vi "eyecat MAX v2_JS.vi"() -> ()   [LabVIEW 2014]
doc: "This VI is an upgrade from the WIN 1_v4 that implements the ageing subrutine"
uses:
  <vilib>/Utility/file.llb/Write To Spreadsheet File (string).vi
  <vilib>/Utility/file.llb/Read From Spreadsheet File (string).vi
  <vilib>/regexp/Match Regular Expression.xnode
  Controls Win/Control 3.ctl
  <vilib>/Utility/miscctls.llb/LVRowAndColumnTypeDef.ctl
  <vilib>/Platform/TimedLoop/XDataNode/XDataNode.xnode
  <vilib>/Platform/TimedLoop/XDataNode/nitl_modes.ctl
  <vilib>/Platform/TimedLoop/XDataNode/XDNodeRunTimeDep.lvlib
  <vilib>/Platform/TimedLoop/XDataNode/wakeup.ctl
  <vilib>/Platform/TimedLoop/XDataNode/timing_clust.ctl
  Buttons/Numeric control.ctl
  <vilib>/Utility/file.llb/Read From Spreadsheet File (DBL).vi
  Buttons/String input.ctl
  Buttons/Numeric indicator.ctl
  Buttons/String output.ctl
panel:
  in  "7170 Override":bool
  out "NO":dbl[](array[numeric])
  out "CO":dbl[](array[numeric])
  out "MKS":bool
  out "7170":bool
  out "Pressure":dbl
  in  "Duration -1":i32
  in  "Demo Sync":i32
  in  "Demo On":bool
  in  "FlowGuide":bool
  in  "Mean(Off)/Interval(On) 2":bool
  in  "Flow Band %":dbl=1.04
  in  "Flow Sync":i32
  in  "Execute Leak Test Button":bool
  out "Emissions":dbl[](array[numeric])
  in  "Temperature Sync":i32
  in  "TempGuide":bool
  in  "Temp Band %":dbl=1.04
  in  "Mean(Off)/Interval(On)":bool
  in  "MKS 5Hz":bool
  out "output cluster":T2
  out "Lambda":dbl[](array[numeric])
  out "MKS HC":dbl
  in  "HC Index":i32
  in  "MFC Number":i32
  out "Open/Closed \nLoop":dbl[](array[numeric])
  out "Air Cyc 2":dbl[](array[numeric])
  in  "Cycle size":i32
  out "MFC Setpoint/Delivery":dynamicdata(graph)
  out "ExtAnDn":bool
  out "ExtAnUp":bool
  out "HC Cyc 2":dbl[](array[numeric])
  out "SO Valve 2":dbl[](array[numeric])
  out "SO Valve 1":dbl[](array[numeric])
  out "Air Bal":dbl[](array[numeric])
  out "HC Bal":dbl[](array[numeric])
  out "Air Cyc 1":dbl[](array[numeric])
  out "HC Cyc 1":dbl[](array[numeric])
  out "File name":string
  out "Log?":bool
  out "Advanced Logging":bool
  out "Connected":bool
  out "Furnace temp 2":dbl
  out "Full system?":bool
  out "Log interval (seconds)":T1
  in  "Flow rate Age":dbl
  in  "Inlet temp Age":dbl
  out "Stopped?":bool
  in  "Stop Cmd":T1
  out "Connected?":bool
  out "Error":dbl
  out "Iteration Duration":i64
  out "Finished Late? [i-1]":bool
  out "Furnace temp 1":dbl
  out "stop 2":bool
  in  "Enum 1":i16=1
  in  "Acknowledge":bool
  out "Test number":u16
  out "Flag1":bool=TRUE
  out "EditPos Subc":T3
  out "Flag 2":bool=TRUE
  in  "Tab Control":T4(tab)
  in  "Leak Test":bool
  in  "Stop Test":bool
  in  "Log Test Data":bool
  in  "Start Test":bool
  in  "Adv Settings":bool
  out "Doors Unlocked":bool
  in  "Temperature Limit (°C)":T1=800.0 min=0.0 max=1200.0 step=1.0
  in  "File Name":T5="Test"
  in  "File Path":path=path "C:/DATA LOG"
  out "Fail":bool
  out "Pass":bool
  in  "Select Test Type":T6(radio)
  out "Standby":bool
  out "Doors Open":bool
  out "Extractor Fan On":bool
  out "Test In Progress":bool
  out "Cool Down":bool
  out "System Alarm":bool
  in  "Inlet Temperature (°C)":T1=400.0 min=350.0 max=1000.0 step=1.0
  in  "Inlet LAMBDA Rich":T1=0.9 min=0.85 max=0.96 step=0.001
  in  "Inlet LAMBDA Lean":T1=1.2 min=1.02 max=3.0 step=0.001
  in  "Test Stop temperature (°C)":T1=300.0 min=100.0 max=1000.0 step=1.0
  in  "Test Start Temperature (°C)":T1=125.0 min=0.0 max=500.0 step=1.0
  in  "Furnace Ramp Rate (°C/min)":T1=15.0 min=1.0 max=50.0 step=0.1
  in  "NO:CO Ratio":T1=1.1 min=1.0 max=5.0 step=0.1
  in  "Inlet O2 (%)":T1=0.5 min=0.0 max=14.0 step=0.01
  in  "Inlet LAMBDA":T1=1.0 min=0.6 max=3.0 step=0.001
  out "Space Velocity (h-1)":T7
  out "Vol Flow @ STP (l/min)":T7
  in  "Test Flow Rate(g/s)":T1 min=0.0 max=100.0 step=0.01
  out "Sample Volume (litres)":T7
  in  "Number of Samples":T1=1.0 min=1.0 max=6.0 step=1.0
  in  "Sample Diameter (mm)":T1
  out "CO Theory (%)":T7 format="%#_3g"
  out "CO Theory (%)":T7 format="%#_3g"
  out "HC Theory (%)":T7
  in  "Sample Length (mm)":T1 min=0.0 step=0.5
  in  "NO ppm SW":dbl=500.0 caption="NO (ppm)" min=0.0 max=500.0 step=1.0
  in  "NO ppm Loff":T1 caption="NO ppm"
  in  "Delete sCycle":bool
  in  "Load sCycle":bool
  in  "Save sCycle":bool
  in  "Clear subcycle":bool
  in  "Clear Cycle Pattern":bool
  in  "Save Cycle":bool
  in  "Load Cycle":bool
  in  "Delete Cycle":bool
  out "Test Compiled":bool
  in  "Compile Test Button":bool
  in  "Sub-Cycle List":i32(listbox)=1
  in  "Cycle List":i32(listbox)=2
  out "Total Test Duration (hrs)":T8
  in  "Ageing Gas":enum32{"Radio Selection 1", "Radio Selection 2"}(radio)
  in  "Sub-Cycle Pattern":string[][](table) caption="Subcycle pattern"
  in  "Total Number of Cycles":T1=1.0 min=1.0 max=10000.0 step=1.0
  in  "Cycle Pattern":string[][](table)
  in  "Sub-Cycle Name":T5
  in  "Cycle Name":T5
  out "Heat Exchanger Temperatures (°C)":dynamicdata(graph)
  out "Flow Rate (g/s)":dynamicdata(graph)
  out "Sample Temperatures (°C)":dynamicdata(graph)
  out "System Temperatures (°C)":dynamicdata(graph)
  out "HC Concentration (ppm)":dynamicdata(graph)
  out "Lambda":dynamicdata(graph)
  out "O2/CO Concentration":dynamicdata(graph)
  out "NO Concentration (ppm)":dynamicdata(graph)
  in  "Purge System":bool
  in  "Alarm ack":bool
  in  "Clear log":bool
  out "Table":string[][](table)
  out "Soft Alarm":bool
  out "Hard Alarm":bool
  # "0 CO \n1 HC Cyc 1\n2 Air Cyc 1\n3 NO\n4 Air Bal\n5 HC Bal\n6 Air Cyc 2\n7 HC Cyc 2"
  # "1% = 0.01"
  # "Test Type"
  # "Test Commands"
  # "System Indicators"
  # "Leak Test"
  # "Catalyst Specification"
  # "Lightoff Settings"
  # "Furnace Lightoff Settings"
  # "Sweep Settings"
  # "CO/HC Lightoff Settings"
  # "0.96 < lambda < 0.85"
  # "1.02< lambda < 1.6"
  # "350 < Tinlet < 1000"
  # "NO Lightoff Settings"
  # "Flow Specification"
  # "Cycle Compiled"
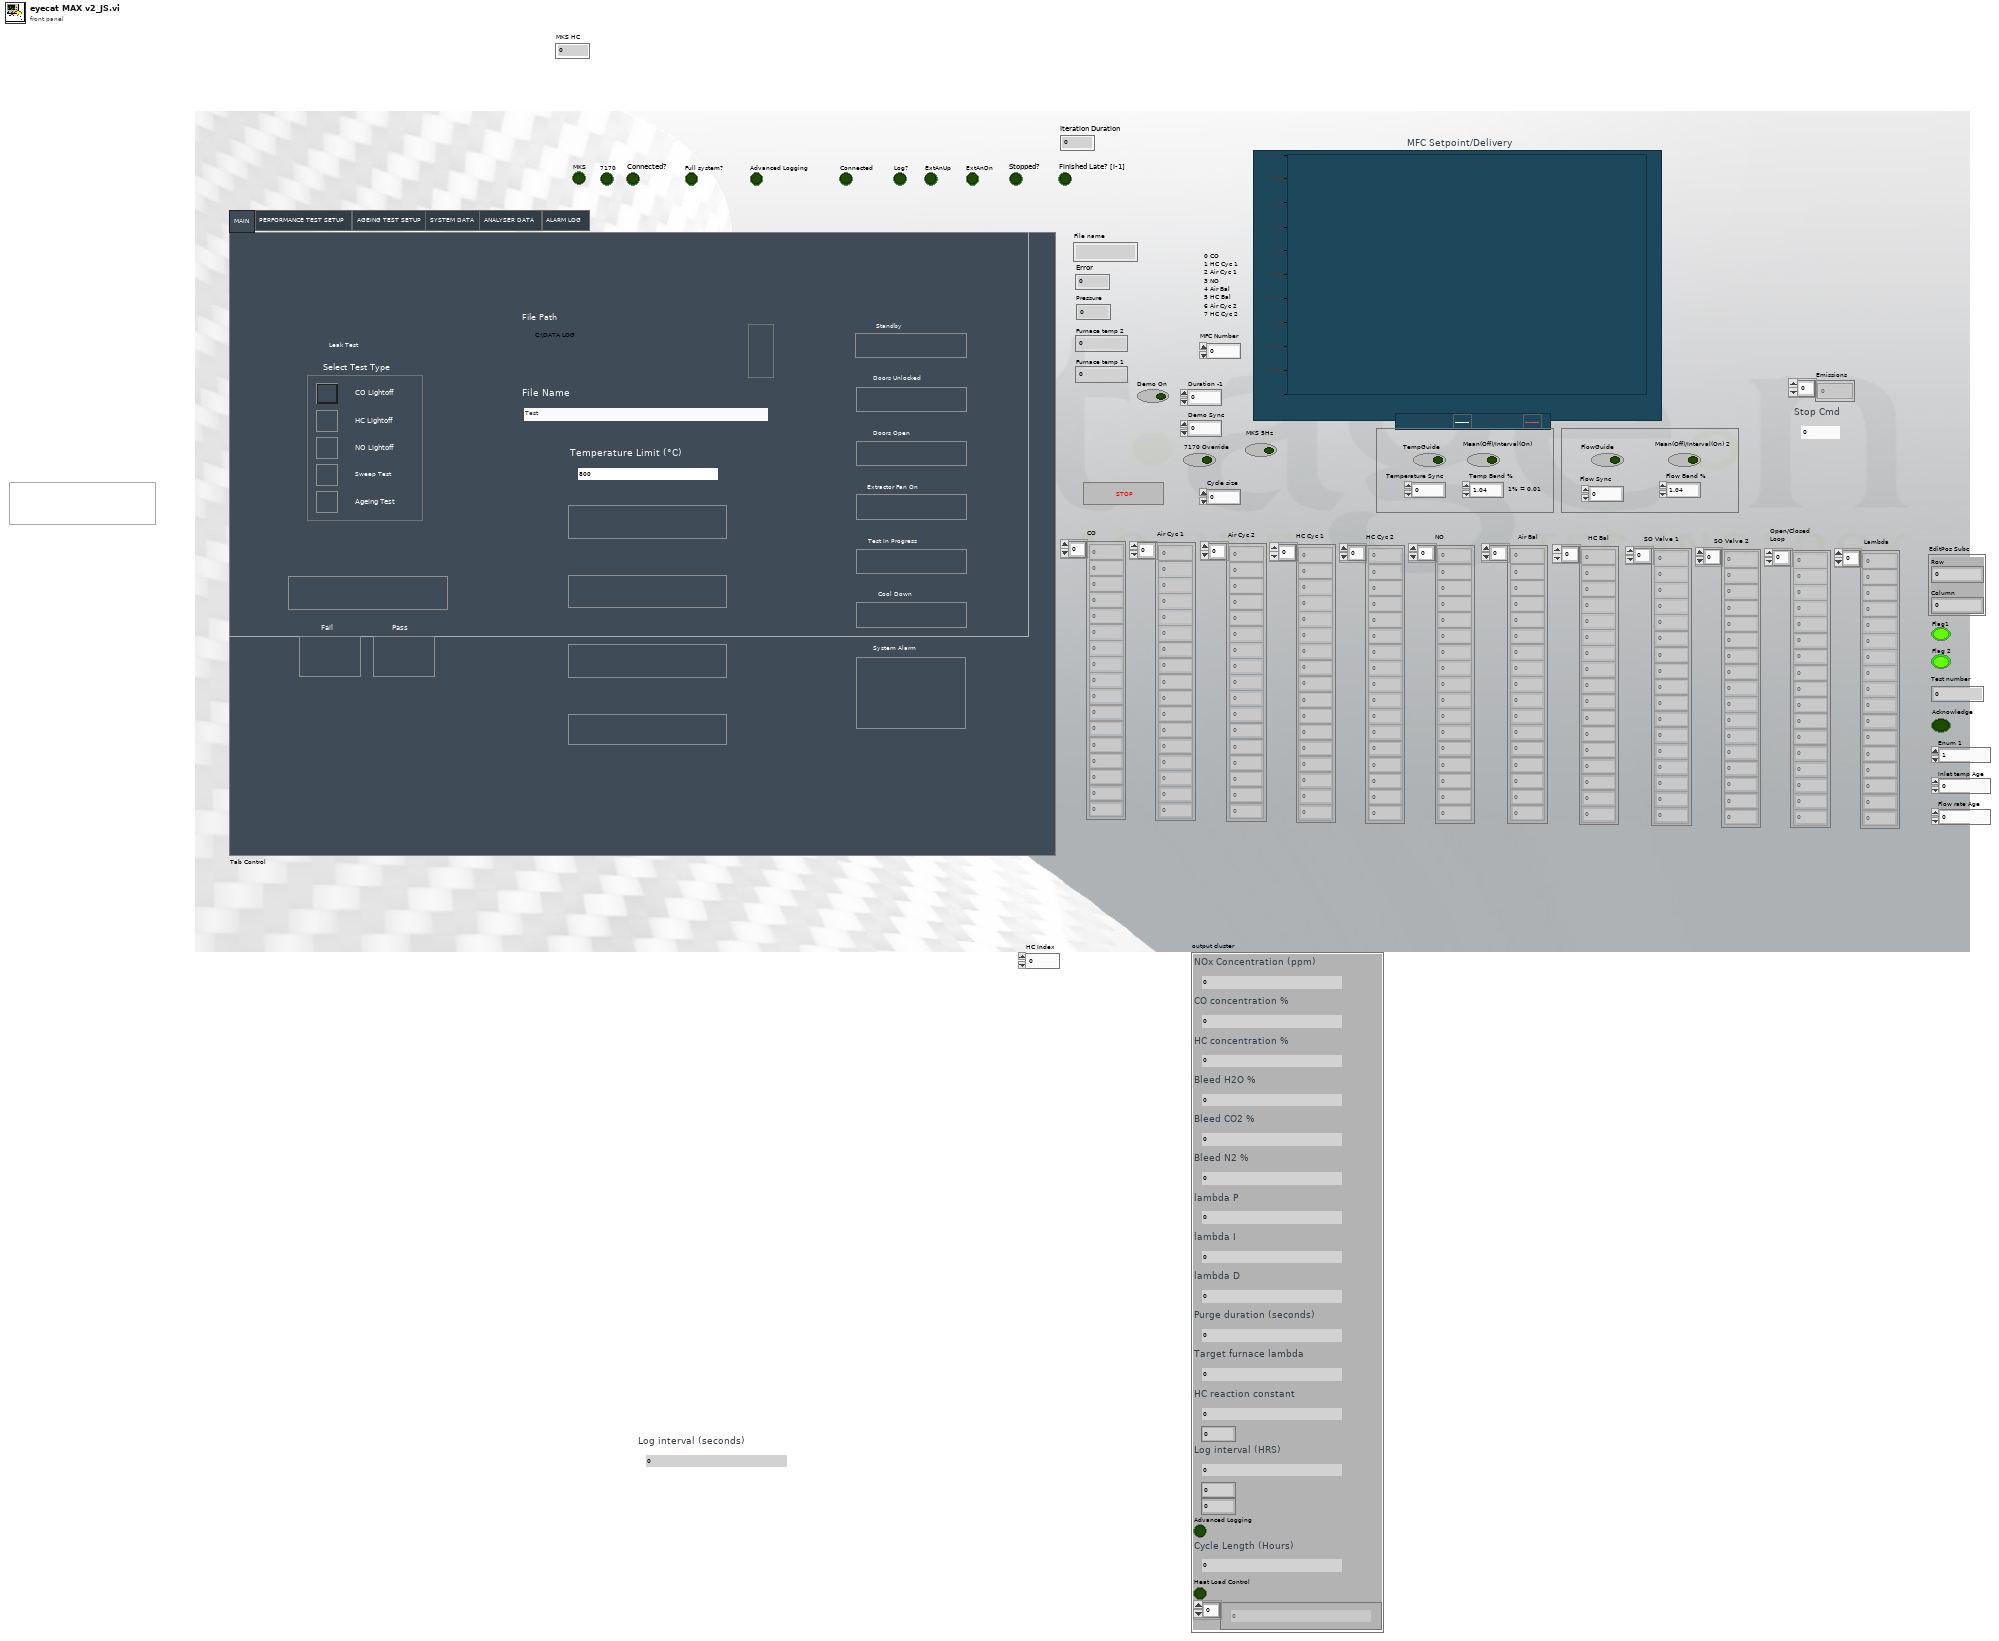
[diagram p1: front panel]
types:
  T1 = typedef "Numeric control.ctl" = dbl
  T2 = cluster{"NOx Concentration (ppm)":T1, "CO concentration %":T1, "HC concentration %":T1, "Bleed H2O %":T1, "Bleed CO2 %":T1, "Bleed N2 %":T1, "lambda P":T1, "lambda I":T1, "lambda D":T1, "Purge duration (seconds)":T1, "Target furnace lambda":T1, "HC reaction constant":T1, i16, "Log interval (HRS)":T1, i16, i16, "Advanced Logging":bool, "Cycle Length (Hours)":T1, "Heat Load Control":bool, T1[]}
  T3 = typedef "LVRowAndColumnTypeDef.ctl" = cluster{"Row":i32, "Column":i32}
  T4 = enum32{"MAIN", "PERFORMANCE TEST SETUP", "AGEING TEST SETUP", "SYSTEM DATA", "ANALYSER DATA", "ALARM LOG"}
  T5 = typedef "String input.ctl" = string
  T6 = enum32{"CO Lightoff", "HC Lightoff", "NO Lightoff", "Sweep Test", "Ageing Test"}
  T7 = typedef "Numeric indicator.ctl" = dbl
  T8 = typedef "String output.ctl" = string
  T9 = typedef "XDNodeRunTimeDep.lvlib/nitl_modes.ctl" = enum32{"No Change", "Process missed periods, maintain original phase", "Discard missed periods, maintain original phase", "Process missed periods, ignore original phase", "Discard missed periods, ignore original phase"}
  T10 = typedef "Control 3.ctl" = enum16{"main", "start test", "save subc", "load subc", "delete subc", "clear table 1", "update list 1", "save cycle", "load cycle", "delete cycle", "clear table 2", "update list 2", "calc HC CO", "Total time calc", "update Cycle pattern ", "load cycle name", "convert to num", "load test array", "check scycle name", "check cycle name", "Multigas connect", "Multigas disconnect", "Leak Test"}
  T11 = enum8{"Enabled", "Disabled", "Disabled and Grayed Out"}
  T12 = typedef "XDNodeRunTimeDep.lvlib/timing_clust.ctl" = cluster{"Expected End [f-1]":u64, "Actual End [f-1]":u64, "Finished Late? [f-1]":bool, "Expected End [i-1]":u64, "Actual End [i-1]":u64, "Finished Late? [i-1]":bool, "Expected Start [i]":u64, "Actual Start [i]":u64, "Expected Start [f]":u64, "Actual Start [f]":u64, "Source Name":string, "Structure Name":string, "Period":i64, "Deadline":i64, "Offset":i64, "Start":i64, "Priority":i32, "Timeout":i32, "Mode":T9, "Wakeup Reason":T13, "Error":errorcluster, "Source Type":string, "Secondary Source Type":string, "Global End Time":u64, "Global Start Time":u64, "Frame Duration":u64, "Iteration Duration":u64, "Assigned CPU":i32, "I/O Scan Engine Mode":u32}
  T13 = typedef "XDNodeRunTimeDep.lvlib/wakeup.ctl" = enum32{"Normal", "Aborted", "Asynchronous wakeup", "Timing source error", "Timed loop error", "Timeout"}
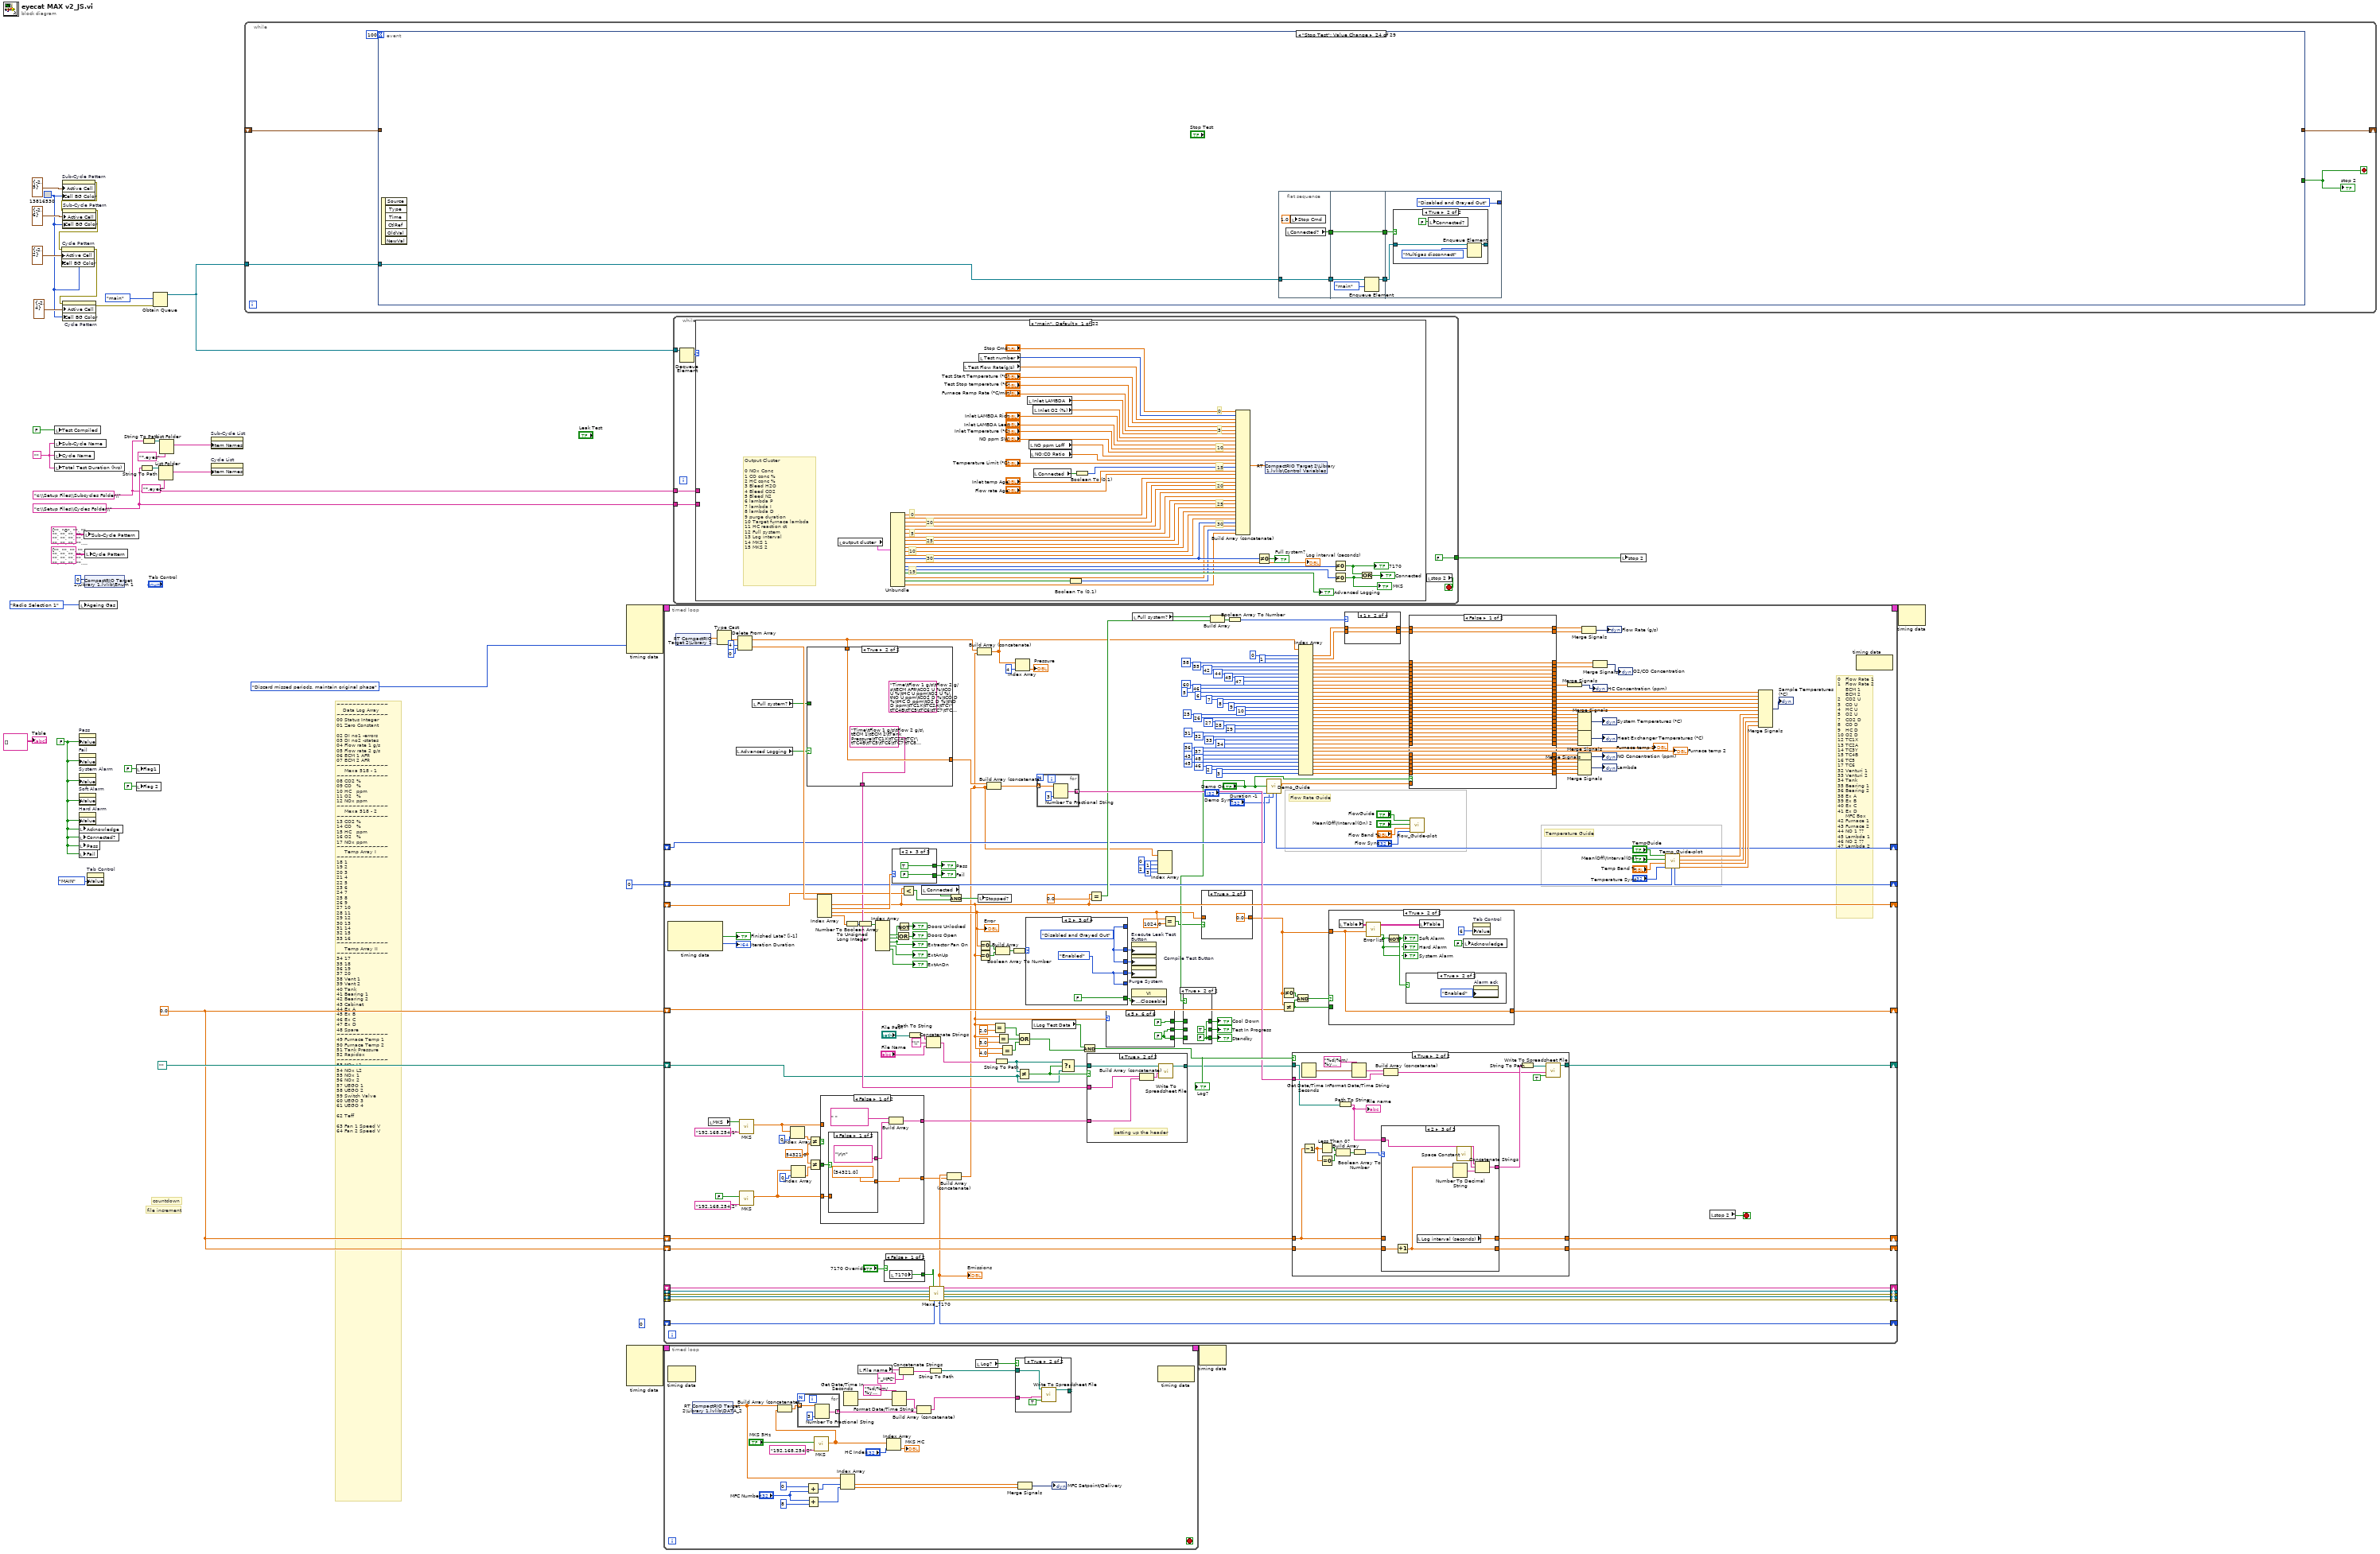
[diagram p0: block diagram]
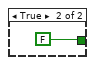
[diagram p3: hidden frame]
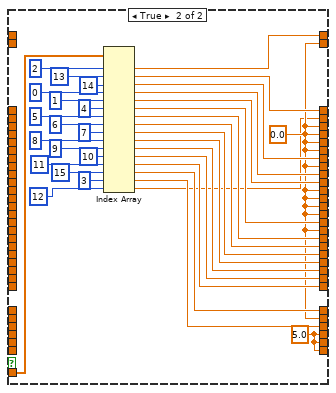
[diagram p6: hidden frame]
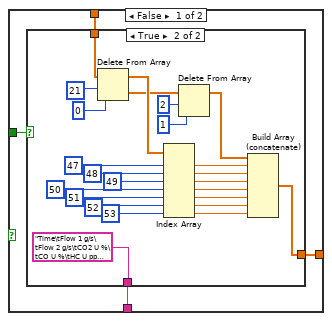
[diagram p7: hidden frame]
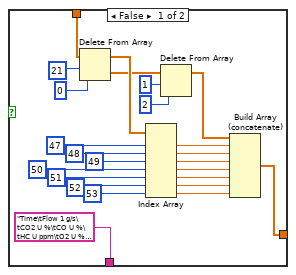
[diagram p8: hidden frame]
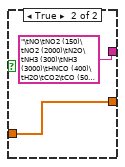
[diagram p9: hidden frame]
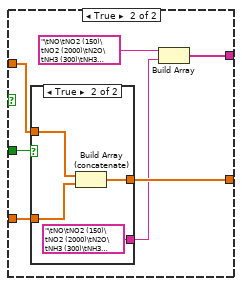
[diagram p10: hidden frame]
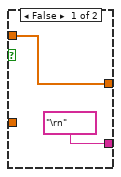
[diagram p11: hidden frame]
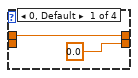
[diagram p12: hidden frame]
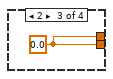
[diagram p13: hidden frame]
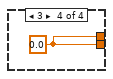
[diagram p14: hidden frame]
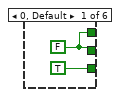
[diagram p15: hidden frame]
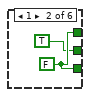
[diagram p16: hidden frame]
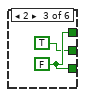
[diagram p17: hidden frame]
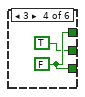
[diagram p18: hidden frame]
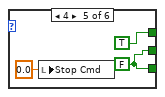
[diagram p19: hidden frame]
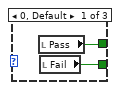
[diagram p20: hidden frame]
diagram:
  (unwired) 0 ("index")
  w5 = FALSE
  w4 = 0.0 ("y")
  w21 = ""
  w24 = "c:\\Setup Files\\Cycles Folder\\"
  w30 = u32 13816530
  w22 = "c:\\Setup Files\\Subcycles Folder\\"
  # "~~~~~~~~~~~~~\n    Data Log Array\n~~~~~~~~~~~~~\n00 Status Integer\n01 Zero Constant\n\n02 DI no1 -errors\n03 DI no2 -states\n04 Flow rate 1 g/s\n05 Flow rate 2 g/s\n06 ECM 1 AFR\n07 ECM 2 AFR\n~~~~~~~~~~~~~\n     Mexa 518 - 1\n~~~~~~~~~~~~~\n08 CO2 %\n09 CO   %\n10 HC   ppm\n11 O2   %\n12 NOx ppm\n~~~~~~~~~~~~~\n     Mexa 518 - 2\n~~~~~~~~~~~~~\n13 CO2 %\n14 CO   %\n15 HC   ppm\n16 O2   %\n17 NOx ppm\n~~~~~~~~~~~~~\n     Temp Array I\n~~~~~~~~~~~~~\n18 1\n19 2 \n20 3\n21 4\n22 5\n23 6\n24 7\n25 8\n26 9\n27 10\n28 11\n29 12\n30 13\n31 14\n32 15\n33 16\n~~~~~~~~~~~~~\n     Temp Array II\n~~~~~~~~~~~~~\n34 17\n35 18\n36 19\n37 20\n38 Vent 1\n39 Vent 2\n40 Tank\n41 Bearing 1\n42 Bearing 2\n43 Cabinet\n44 Ex A\n45 Ex B\n46 Ex C\n47 Ex D\n48 Spare\n~~~~~~~~~~~~~\n49 Furnace Temp 1\n50 Furnace Temp 2\n51 Tank Pressure\n52 Rapidox\n~~~~~~~~~~~~~\n53 NOx L1\n54 NOx L2\n55 NOx 1\n56 NOx 2\n57 UEGO 1\n58 UEGO 2\n59 Switch Valve\n60 UEGO 3\n61 UEGO 4\n\n62 Teff\n\n63 Fan 1 Speed V\n64 Fan 2 Speed V"
  # "file increment"
  # "countdown"
  n1 = local write "Test Compiled"(FALSE ("Cycle Compiled")) -> ()
  n2 = local write "Sub-Cycle Name"(w21) -> ()
  n3 = local write "Cycle Name"(w21) -> ()
  n4 = local write "Total Test Duration (hrs)"(w21) -> ()
  n5 = property on="Sub-Cycle Pattern" class="Tbl (strict)"("Active Cell"=T3 {"Row"=-2, "Column"=5} ("Active Cell:Active Cell"), "Cell BG Color"=w30) -> (error out=w35:errorcluster)  [unwired: 2 in, 1 out]
  n6 = property on="Sub-Cycle Pattern" class="Tbl (strict)"(error in=w35, "Active Cell"=T3 {"Row"=-2, "Column"=6} ("Active Cell:Active Cell"), "Cell BG Color"=w30) -> (error out=w34:errorcluster)  [unwired: 1 in, 1 out]
  n7 = property on="Cycle Pattern" class="Tbl (strict)"(error in=w34, "Active Cell"=T3 {"Row"=-2, "Column"=2} ("Active Cell:Active Cell"), "Cell BG Color"=w30) -> (error out=w32:errorcluster)  [unwired: 1 in, 1 out]
  n8 = property on="Cycle Pattern" class="Tbl (strict)"(error in=w32, "Active Cell"=T3 {"Row"=-2, "Column"=4} ("Active Cell:Active Cell"), "Cell BG Color"=w30) -> (error out=w29:errorcluster)  [unwired: 1 in, 1 out]
  n9 = property on="Pass" class="Bool (strict)"("Value"=w5) -> ()  [unwired: 2 in, 2 out]
  n10 = property on="Fail" class="Bool (strict)"("Value"=w5) -> ()  [unwired: 2 in, 2 out]
  n11 = property on="System Alarm" class="Bool (strict)"("Value"=w5) -> ()  [unwired: 2 in, 2 out]
  n12 = property on="Soft Alarm" class="Bool (strict)"("Value"=w5) -> ()  [unwired: 2 in, 2 out]
  n13 = property on="Hard Alarm" class="Bool (strict)"("Value"=w5) -> ()  [unwired: 2 in, 2 out]
  n14 = local write "Acknowledge"(w5) -> ()
  n15 = local write "Connected?"(w5) -> ()
  n16 = local write "Pass"(w5) -> ()
  n17 = local write "Fail"(w5) -> ()
  n18 = local write "Ageing Gas"(enum32{"Radio Selection 1", "Radio Selection 2"}."Radio Selection 1" ("Ageing Gas")) -> ()
  n19 = local write "Sub-Cycle Pattern"(string[][] [["", "0", "", "", "", "", "", "", "", "", "", "", ""], ["", "", "", "", "", "", "", "", "", "", "", "", ""], ["", "", "", "", "", "", "", "", "", "", "", "", ""], ["", "", "", "", "", "", "", "", "", "", "", "", ""], ["", "", "", "", "", "", "", "", "", "", "", "", ""], ["", "", "", "", "", "", "", "", "", "", "", "", ""], ["", "", "", "", "", "", "", "", "", "", "", "", ""], ["", "", "", "", "", "", "", "", "", "", "", "", ""], ["", "", "", "", "", "", "", "", "", "", "", "", ""], ["", "", "", "", "", "", "", "", "", "", "", "", ""], ["", "", "", "", "", "", "", "", "", "", "", "", ""], ["", "", "", "", "", "", "", "", "", "", "", "", ""], ["", "", "", "", "", "", "", "", "", "", "", "", ""], ["", "", "", "", "", "", "", "", "", "", "", "", ""], ["", "", "", "", "", "", "", "", "", "", "", "", ""], ["", "", "", "", "", "", "", "", "", "", "", "", ""], ["", "", "", "", "", "", "", "", "", "", "", "", ""], ["", "", "", "", "", "", "", "", "", "", "", "", ""], ["", "", "", "", "", "", "", "", "", "", "", "", ""], ["", "", "", "", "", "", "", "", "", "", "", "", ""], ["", "", "", "", "", "", "", "", "", "", "", "", ""], ["", "", "", "", "", "", "", "", "", "", "", "", ""], ["", "", "", "", "", "", "", "", "", "", "", "", ""], ["", "", "", "", "", "", "", "", "", "", "", "", ""], ["", "", "", "", "", "", "", "", "", "", "", "", ""], ["", "", "", "", "", "", "", "", "", "", "", "", ""], ["", "", "", "", "", "", "", "", "", "", "", "", ""], ["", "", "", "", "", "", "", "", "", "", "", "", ""], ["", "", "", "", "", "", "", "", "", "", "", "", ""], ["", "", "", "", "", "", "", "", "", "", "", "", ""], ["", "", "", "", "", "", "", "", "", "", "", "", ""]]) -> ()
  n20 = local write "Cycle Pattern"(string[][] [["", "", "", "", ""], ["", "", "", "", ""], ["", "", "", "", ""], ["", "", "", "", ""], ["", "", "", "", ""], ["", "", "", "", ""], ["", "", "", "", ""], ["", "", "", "", ""], ["", "", "", "", ""], ["", "", "", "", ""], ["", "", "", "", ""], ["", "", "", "", ""], ["", "", "", "", ""], ["", "", "", "", ""], ["", "", "", "", ""], ["", "", "", "", ""], ["", "", "", "", ""], ["", "", "", "", ""], ["", "", "", "", ""], ["", "", "", "", ""], ["", "", "", "", ""], ["", "", "", "", ""], ["", "", "", "", ""], ["", "", "", "", ""], ["", "", "", "", ""], ["", "", "", "", ""], ["", "", "", "", ""], ["", "", "", "", ""], ["", "", "", "", ""], ["", "", "", "", ""], ["", "", "", "", ""]]) -> ()
  n21 = shared-variable "RT CompactRIO Target 2\\Library 1.lvlib\\Enum 1"(u16 0 ("Enum 1")) -> ()  [unwired: 1 in, 1 out]
  n22 = property on="Tab Control" class="TabCtl (strict)"("Value"=T4."MAIN" ("Tab Control")) -> ()  [unwired: 2 in, 2 out]
  n23 = local write "Flag1"(FALSE) -> ()
  n24 = local write "Flag 2"(FALSE) -> ()
  n25 = String To Path(string=w24) -> (path=w25:path)
  n26 = String To Path(string=w22) -> (path=w27:path)
  n27 = Obtain Queue(element data type=Control_3."main" ("Enum"), error in (no error)=w29) -> (queue out=w38:refnum<queue>)  [unwired: 3 in, 2 out]
  n28 = List Folder(path=w25, pattern="*.eyec") -> (filenames=w26:string[])  [unwired: 2 in, 3 out]
  n29 = List Folder(path=w27, pattern="*.eyes") -> (filenames=w28:string[])  [unwired: 2 in, 3 out]
  n30 = property on="Sub-Cycle List" class="LstBox (strict)"("Item Names"=w28) -> ()  [unwired: 2 in, 2 out]
  n31 = property on="Cycle List" class="LstBox (strict)"("Item Names"=w26) -> ()  [unwired: 2 in, 2 out]
  n32 = while {
    tunnel: w38 -> [w44]
    shift-right: [w42] -> _
    shift-left: _ -> [w41]
    stop <- w40 stop-if-true
    n33 = event shown="[23] \"Stop Test\": Value Change" {
      selector: _ -> [_ _ _ _ _ _ _ _ _ _ _ _ _ _ _ _ _ _ _ _ _ _ _ _ _ _ _ _ _]
      dyn-events: _ -> [_ _ _ _ _ _ _ _ _ _ _ _ _ _ _ _ _ _ _ _ _ _ _ _ _ _ _ _ _]
      timeout: 100 -> [_ _ _ _ _ _ _ _ _ _ _ _ _ _ _ _ _ _ _ _ _ _ _ _ _ _ _ _ _]
      tunnel: w44 -> [w47 w49 _ w58 w66 w73 w80 w91 w95 w106 w111 w114 w119 w141 w149 w150 _ _ _ _ w195 w211 _ w297 w315 _ w329 _ _]
      tunnel: [w45 w48 _ w59 w65 w72 w79 w90 w93 w101 w108 w113 w117 w138 _ _ _ _ _ _ _ _ _ _ _ _ _ _ _] -> w42
      tunnel: w41 -> [w45 w48 _ w59 w65 w72 w78 w90 w93 w101 w108 w113 w117 w138 _ _ _ _ _ _ _ _ _ _ _ _ _ _ _]
      tunnel: [_ _ w51 _ _ _ _ _ _ _ _ _ _ _ _ _ _ _ _ _ _ _ _ _ _ _ _ _ _] -> w40
      event Timeout {
        n34 = event-data() -> ()  [unwired: 1 in, 2 out]
        n35 = Enqueue Element(queue=w47, element=Control_3."main" ("Enum")) -> ()  [unwired: 2 in, 3 out]
      }
      event "Clear subcycle": Value Change {
        n36 = event-data() -> ()  [unwired: 1 in, 5 out]
        n37 = Enqueue Element(queue=w49, element=Control_3."clear table 1" ("Enum")) -> ()  [unwired: 2 in, 3 out]
      }
      event Panel Close? {
        n38 = event-data() -> ()  [unwired: 1 in, 3 out]
        n39 = Two Button Dialog(message="This command will close Eyecat!\nDo you wish to continue?", 1:"No" ("F button name (\"Cancel\")"), 2:"Yes" ("T button name (\"OK\")")) -> (T button?=w51:bool)
        n40 = Not(x=w51) -> (.not. x?=w52:bool)
        n41 = event-data("Discard?"=w52) -> ()  [unwired: 1 in, 1 out]
      }
      event "Save sCycle": Value Change {
        n42 = event-data() -> ()  [unwired: 1 in, 5 out]
        n43 = local read "Sub-Cycle Pattern"() -> (w56:string[][])
        n44 = call "Time column check.vi"("Array"=w56) -> ("Mistake?"=w57:bool)  [unwired: 10 in]
        n45 = case shown="False" w57 {
          tunnel: w58 -> [w60 _]
          frame False {
            n46 = Enqueue Element(queue=w60, element=Control_3."save subc") -> (queue out=w62:refnum<queue>)  [unwired: 2 in, 2 out]
            n47 = Enqueue Element(queue=w62, element=Control_3."update list 1") -> ()  [unwired: 2 in, 3 out]
          }
          frame True {
            n48 = One Button Dialog(message="The time sequence is incorrect!\nReview and save again!") -> ()  [unwired: 1 in, 1 out]
          }
        }
      }
      event "Load sCycle": Value Change {
        n49 = event-data() -> ()  [unwired: 1 in, 5 out]
        n50 = Enqueue Element(queue=w66, element=Control_3."load subc") -> ()  [unwired: 2 in, 3 out]
      }
      event "Delete sCycle": Value Change {
        n51 = event-data() -> ()  [unwired: 1 in, 5 out]
        n52 = Enqueue Element(queue=w73, element=Control_3."delete subc") -> (queue out=w75:refnum<queue>)  [unwired: 2 in, 2 out]
        n53 = Enqueue Element(queue=w75, element=Control_3."update list 1") -> (queue out=w71:refnum<queue>)  [unwired: 2 in, 2 out]
        n54 = Enqueue Element(queue=w71, element=Control_3."update Cycle pattern ") -> (queue out=w68:refnum<queue>)  [unwired: 2 in, 2 out]
        n55 = Enqueue Element(queue=w68, element=Control_3."Total time calc") -> ()  [unwired: 2 in, 3 out]
      }
      event "Sub-Cycle Pattern": Mouse Down; "Sub-Cycle Pattern": Value Change {
        n56 = event-data() -> ()  [unwired: 1 in, 3 out]
        n57 = property on="Sub-Cycle Pattern" class="Tbl (strict)"() -> ("EditPos"=w79:T3)  [unwired: 2 in, 2 out]
        n58 = Unbundle By Name(w79) -> ("Row"=w81:i32)  [unwired: 1 out]
        n59 = Less?(x=w81, y=30) -> (x < y?=w83:bool)
        n60 = case shown="True" w83 {
          tunnel: w80 -> [_ w88]
          frame False {
            n61 = One Button Dialog(message="This table is limited to 30 entries!") -> ()  [unwired: 1 in, 1 out]
          }
          frame True {
            n62 = Enqueue Element(queue=w88, element=Control_3."convert to num") -> (queue out=w87:refnum<queue>)  [unwired: 2 in, 2 out]
            n63 = Enqueue Element(queue=w87, element=Control_3."calc HC CO") -> ()  [unwired: 2 in, 3 out]
          }
        }
        "EditPos Subc" <- w78
        "Flag1" <- TRUE
      }
      event "Clear Cycle Pattern": Value Change {
        n64 = event-data() -> ()  [unwired: 1 in, 5 out]
        n65 = Enqueue Element(queue=w91, element=Control_3."clear table 2" ("Enum")) -> ()  [unwired: 2 in, 3 out]
        n66 = local write "Test Compiled"(FALSE ("Test Compiled")) -> ()
      }
      event "Save Cycle": Value Change {
        n67 = event-data() -> ()  [unwired: 1 in, 5 out]
        n68 = Enqueue Element(queue=w95, element=Control_3."update Cycle pattern ") -> (queue out=w94:refnum<queue>)  [unwired: 2 in, 2 out]
        n69 = Enqueue Element(queue=w94, element=Control_3."save cycle") -> (queue out=w98:refnum<queue>)  [unwired: 2 in, 2 out]
        n70 = Enqueue Element(queue=w98, element=Control_3."update list 2") -> ()  [unwired: 2 in, 3 out]
      }
      event "Load Cycle": Value Change {
        n71 = event-data() -> ()  [unwired: 1 in, 5 out]
        n72 = Enqueue Element(queue=w106, element=Control_3."load cycle") -> (queue out=w104:refnum<queue>)  [unwired: 2 in, 2 out]
        n73 = Enqueue Element(queue=w104, element=Control_3."update Cycle pattern ") -> (queue out=w103:refnum<queue>)  [unwired: 2 in, 2 out]
        n74 = local write "Test Compiled"(FALSE ("Test Compiled")) -> ()
        n75 = Enqueue Element(queue=w103, element=Control_3."Total time calc") -> ()  [unwired: 2 in, 3 out]
      }
      event "Delete Cycle": Value Change {
        n76 = event-data() -> ()  [unwired: 1 in, 5 out]
        n77 = Enqueue Element(queue=w111, element=Control_3."delete cycle") -> (queue out=w110:refnum<queue>)  [unwired: 2 in, 2 out]
        n78 = Enqueue Element(queue=w110, element=Control_3."update list 2") -> ()  [unwired: 2 in, 3 out]
      }
      event Value Change {
        n79 = event-data() -> ()  [unwired: 1 in, 5 out]
        n80 = Enqueue Element(queue=w114, element=Control_3."Total time calc") -> ()  [unwired: 2 in, 3 out]
      }
      event "Cycle Pattern": Mouse Up; "Cycle Pattern": Value Change {
        n81 = event-data() -> ()  [unwired: 1 in, 3 out]
        n82 = property on="Cycle Pattern" class="Tbl (strict)"() -> ("EditPos"=w121:T3)  [unwired: 2 in, 2 out]
        n83 = Unbundle By Name(w121) -> ("Row"=w118:i32, "Column"=w123:i32)
        n84 = Less?(x=w118, y=30) -> (x < y?=w122:bool)
        n85 = case shown="True" w122 {
          tunnel: w123 -> [_ w125]
          tunnel: w119 -> [_ w128]
          frame False {
            n86 = One Button Dialog(message="This table is limited to 30 entries!") -> ()  [unwired: 1 in, 1 out]
          }
          frame True {
            n87 = Equal?(x=w125, y=1) -> (x = y?=w129:bool)
            n88 = case shown="True" w129 {
              tunnel: w128 -> [w132 w135]
              tunnel: [w131 w134] -> w127
              frame False {
                n89 = Enqueue Element(queue=w132, element=Control_3."update Cycle pattern ") -> (queue out=w131:refnum<queue>)  [unwired: 2 in, 2 out]
              }
              frame True {
                n90 = Enqueue Element(queue=w135, element=Control_3."load cycle name") -> (queue out=w134:refnum<queue>)  [unwired: 2 in, 2 out]
              }
            }
            n91 = Enqueue Element(queue=w127, element=Control_3."Total time calc") -> ()  [unwired: 2 in, 3 out]
          }
        }
        "Flag 2" <- TRUE
      }
      event "Compile Test Button": Value Change {
        n92 = event-data() -> ()  [unwired: 1 in, 5 out]
        n93 = local read "Flag 2"() -> (w137:bool)
        n94 = case shown="True" w137 {
          tunnel: w141 -> [w142 w146]
          tunnel: [w142 w143] -> w139
          frame False {
          }
          frame True {
            n95 = Enqueue Element(queue=w146, element=Control_3."save cycle") -> (queue out=w144:refnum<queue>)  [unwired: 2 in, 2 out]
            n96 = Enqueue Element(queue=w144, element=Control_3."update list 2") -> (queue out=w143:refnum<queue>)  [unwired: 2 in, 2 out]
          }
        }
        n97 = Enqueue Element(queue=w139, element=Control_3."load test array") -> ()  [unwired: 2 in, 3 out]
      }
      event Value Change {
        n98 = event-data() -> ()  [unwired: 1 in, 5 out]
        n99 = Enqueue Element(queue=w149, element=Control_3."check scycle name") -> ()  [unwired: 2 in, 3 out]
      }
      event Value Change {
        n100 = event-data() -> ()  [unwired: 1 in, 5 out]
        n101 = Enqueue Element(queue=w150, element=Control_3."check cycle name") -> ()  [unwired: 2 in, 3 out]
      }
      event Value Change {
        n102 = event-data() -> ()  [unwired: 1 in, 5 out]
        n103 = Square(x="Sample Diameter (mm)") -> (x^2=w159:T1)
        n104 = Compound Arithmetic op=MULTIPLY(w159, "Sample Length (mm)", "Number of Samples", 3.141592653589793) -> (w158:T1)
        n105 = Divide(x=w158, y=4000000.0) -> (x/y=→"Sample Volume (litres)":T1)
      }
      event Value Change {
        # "O2Eq"
        n106 = event-data() -> ()  [unwired: 1 in, 5 out]
        n107 = local write "Inlet LAMBDA"("Inlet LAMBDA") -> ()
        n108 = local write "Inlet O2 (%)"("Inlet O2 (%)") -> ()
        n109 = Decrement(x="Inlet LAMBDA") -> (x-1=w174:T1)
        n110 = Multiply(x=4.76, y="Inlet LAMBDA") -> (x*y=w170:T1)
        n111 = Multiply(x=w174, y=100.0) -> (x*y=w172:T1)
        n112 = Add(x=0.33, y=w170) -> (x+y=w168:T1)
        n113 = Divide(x=w172, y=w168) -> (x/y=w167:T1)
        n114 = Subtract(x="Inlet O2 (%)", y=w167) -> (x-y=w165:T1)
        n115 = Multiply(x=w165, y=2.0) -> (x*y=→"CO Theory (%)":T1)
        n116 = Divide(x=w165, y=4.5) -> (x/y=→"HC Theory (%)":T1)
      }
      event Value Change {
        n117 = event-data() -> ()  [unwired: 1 in, 5 out]
        n118 = local write "NO ppm Loff"("NO ppm Loff") -> ()
        n119 = local write "NO:CO Ratio"("NO:CO Ratio") -> ()
        n120 = Divide(x="NO ppm Loff", y=T1 10000.0) -> (x/y=w177:T1)
        n121 = Multiply(x="NO:CO Ratio", y=w177) -> (x*y=→"CO Theory (%)":T1)
      }
      event Value Change {
        n122 = event-data() -> ()  [unwired: 1 in, 5 out]
        n123 = local read "Sample Volume (litres)"() -> (w182:T7)
        n124 = Equal?(x=w182, y=0.0) -> (x = y?=w181:bool)
        n125 = case shown="False" w181 {
          tunnel: w182 -> [w187 _]
          tunnel: "Test Flow Rate(g/s)" -> [w184 _]
          frame False {
            w189 = 60.0 ("y")
            n126 = Multiply(x=w184, y=w189) -> (x*y=w191:T1)
            n127 = Divide(x=w191, y=1.2) -> (x/y=w186:T1)
            "Vol Flow @ STP (l/min)" <- w186
            n128 = Multiply(x=w186, y=w189) -> (x*y=w188:T1)
            n129 = Divide(x=w188, y=w187) -> (x/y=→"Space Velocity (h-1)":T1)
          }
          frame True {
            n130 = One Button Dialog(message="Review sample specification first!") -> ()  [unwired: 1 in, 1 out]
          }
        }
      }
      event "Execute Leak Test Button": Value Change {
        n131 = event-data() -> ()  [unwired: 1 in, 5 out]
        n132 = flat-sequence {
          tunnel: w195 -> [w198]
          tunnel: [w198] -> w194
          tunnel: w194 -> [w201]
          frame #0 {
            n133 = local write "Test number"(u16 5) -> ()
            n134 = local write "Enum 1"(u16 3 ("Test number")) -> ()
          }
          frame #1 {
            n135 = Enqueue Element(queue=w201, element=Control_3."main" ("Enum")) -> (queue out=w199:refnum<queue>)  [unwired: 2 in, 2 out]
            n136 = Enqueue Element(queue=w199, element=Control_3."start test" ("Enum")) -> ()  [unwired: 2 in, 3 out]
          }
        }
        n137 = local read "Pressure"() -> (w193:dbl)
        n138 = call "Press_Test.vi"(10:w193) -> ()  [unwired: 10 in, 1 out]
      }
      event "Start Test": Value Change {
        n139 = event-data() -> ()  [unwired: 1 in, 6 out]
        n140 = local read "Log Test Data"() -> (w203:bool)
        n141 = Boolean To (0,1)(Boolean=w203) -> (0, 1=w210:i16)
        n142 = Equal To 0?(x=w210) -> (x = 0?=w209:bool)
        n143 = case shown="True" w209 {
          tunnel: [TRUE ("T button?") w275] -> w204
          frame False {
          }
          frame True {
            # "Log Data Check"
            n144 = Two Button Dialog(message="You are not currently logging data!\nDo you wish to continue?", 1:"No" ("T button name (\"OK\")"), 2:"Yes" ("T button name (\"OK\")")) -> (T button?=w275:bool)
          }
        }
        n145 = Equal?(x=2.0, y=2.0) -> (x = y?=w205:bool)
        n146 = And(x=w205, y=w204) -> (x .and. y?=w206:bool)
        n147 = case shown="True" w206 {
          frame False {
          }
          frame True {
            n148 = flat-sequence {
              tunnel: "Cycle size" -> [w225]
              tunnel: [w225] -> w214
              tunnel: [w228] -> w223
              tunnel: w214 -> [w228]
              tunnel: w223 -> [w231]
              tunnel: [w231] -> w222
              tunnel: w222 -> [w234]
              tunnel: [w234] -> w221
              tunnel: w221 -> [w237]
              tunnel: [w237] -> w213
              tunnel: w213 -> [w240]
              tunnel: [w240] -> w212
              tunnel: [w243] -> w224
              tunnel: w212 -> [w243]
              tunnel: [w246] -> w220
              tunnel: w224 -> [w246]
              tunnel: w220 -> [w249]
              tunnel: [w249] -> w218
              tunnel: w218 -> [w252]
              tunnel: [w252] -> w217
              tunnel: w217 -> [w255]
              tunnel: [w255] -> w216
              tunnel: w216 -> [w261]
              tunnel: [w261] -> w215
              tunnel: w215 -> [w272]
              frame #0 {
                n149 = call-poly <vilib>:"Read From Spreadsheet File.vi"() -> ("all rows"=w226:dbl[][])  [unwired: 7 in, 4 out]
                n150 = Reshape Array(w226, w225) -> (→"CO":dbl[])
              }
              frame #1 {
                n151 = call-poly <vilib>:"Read From Spreadsheet File.vi"() -> ("all rows"=w230:dbl[][])  [unwired: 7 in, 4 out]
                n152 = Reshape Array(w230, w228) -> (→"Air Cyc 1":dbl[])
              }
              frame #2 {
                n153 = call-poly <vilib>:"Read From Spreadsheet File.vi"() -> ("all rows"=w232:dbl[][])  [unwired: 7 in, 4 out]
                n154 = Reshape Array(w232, w231) -> (→"Air Cyc 2":dbl[])
              }
              frame #3 {
                n155 = call-poly <vilib>:"Read From Spreadsheet File.vi"() -> ("all rows"=w236:dbl[][])  [unwired: 7 in, 4 out]
                n156 = Reshape Array(w236, w234) -> (→"HC Cyc 1":dbl[])
              }
              frame #4 {
                n157 = call-poly <vilib>:"Read From Spreadsheet File.vi"() -> ("all rows"=w239:dbl[][])  [unwired: 7 in, 4 out]
                n158 = Reshape Array(w239, w237) -> (→"HC Cyc 2":dbl[])
              }
              frame #5 {
                n159 = call-poly <vilib>:"Read From Spreadsheet File.vi"() -> ("all rows"=w241:dbl[][])  [unwired: 7 in, 4 out]
                n160 = Reshape Array(w241, w240) -> (→"NO":dbl[])
              }
              frame #6 {
                n161 = call-poly <vilib>:"Read From Spreadsheet File.vi"() -> ("all rows"=w244:dbl[][])  [unwired: 7 in, 4 out]
                n162 = Reshape Array(w244, w243) -> (→"Air Bal":dbl[])
              }
              frame #7 {
                n163 = call-poly <vilib>:"Read From Spreadsheet File.vi"() -> ("all rows"=w248:dbl[][])  [unwired: 7 in, 4 out]
                n164 = Reshape Array(w248, w246) -> (→"HC Bal":dbl[])
              }
              frame #8 {
                n165 = call-poly <vilib>:"Read From Spreadsheet File.vi"() -> ("all rows"=w250:dbl[][])  [unwired: 7 in, 4 out]
                n166 = Reshape Array(w250, w249) -> (→"SO Valve 1":dbl[])
              }
              frame #9 {
                n167 = call-poly <vilib>:"Read From Spreadsheet File.vi"() -> ("all rows"=w253:dbl[][])  [unwired: 7 in, 4 out]
                n168 = Reshape Array(w253, w252) -> (→"SO Valve 2":dbl[])
              }
              frame #10 {
                n169 = call-poly <vilib>:"Read From Spreadsheet File.vi"() -> ("all rows"=w257:dbl[][])  [unwired: 7 in, 4 out]
                n170 = Reshape Array(w257, w255) -> (→"Open/Closed \nLoop":dbl[])
              }
              frame #11 {
                n171 = local read "Open/Closed \nLoop"() -> (w262:dbl[])
                n172 = local read "SO Valve 1"() -> (w264:dbl[])
                n173 = local read "SO Valve 2"() -> (w263:dbl[])
                n174 = local read "HC Cyc 2"() -> (w267:dbl[])
                n175 = local read "HC Cyc 1"() -> (w266:dbl[])
                n176 = local read "Air Cyc 1"() -> (w260:dbl[])
                n177 = local read "Air Cyc 2"() -> (w265:dbl[])
                n178 = local read "HC Bal"() -> (w269:dbl[])
                n179 = local read "Air Bal"() -> (w268:dbl[])
                n180 = local read "NO"() -> (w258:dbl[])
                n181 = local read "CO"() -> (w259:dbl[])
                n182 = Build Array (concatenate)(w261, w259, w260, w265, w266, w267, w258, w268, w269, w264, w263, w262) -> (w270:dbl[])
                n183 = shared-variable "RT CompactRIO Target 2\\Library 1.lvlib\\Inject_Arrays"(w270) -> ()  [unwired: 1 in, 1 out]
              }
              frame #12 {
                n184 = call-poly <vilib>:"Read From Spreadsheet File.vi"() -> ("all rows"=w273:dbl[][])  [unwired: 7 in, 4 out]
                n185 = Reshape Array(w273, w272) -> (w271:dbl[])
                "Lambda" <- w271
                n186 = shared-variable "RT CompactRIO Target 2\\Library 1.lvlib\\Inject_Arrays_Lambda"(w271) -> ()  [unwired: 1 in, 1 out]
              }
            }
          }
        }
        n187 = case shown="True" w204 {
          tunnel: w211 -> [_ w280]
          frame False {
          }
          frame True {
            n188 = flat-sequence {
              tunnel: w280 -> [w283]
              tunnel: [w283] -> w279
              tunnel: w279 -> [w287]
              frame #0 {
                n189 = local write "Enum 1"(u16 1 ("Test number")) -> ()
                "Test number" <- "Select Test Type"
              }
              frame #1 {
                n190 = Enqueue Element(queue=w287, element=Control_3."main" ("Enum")) -> (queue out=w285:refnum<queue>)  [unwired: 2 in, 2 out]
                n191 = property on="Stop Test" class="Bool (strict)"("DisabledEnum"=T11."Enabled" ("Disabled")) -> ()  [unwired: 2 in, 2 out]
                n192 = Enqueue Element(queue=w285, element=Control_3."start test" ("Enum")) -> ()  [unwired: 2 in, 3 out]
              }
            }
          }
        }
      }
      event "Log Test Data": Value Change {
        n193 = event-data() -> ()  [unwired: 1 in, 6 out]
        n194 = property on="File Name" class="Str (strict)"() -> ("Value"=w291:T5)  [unwired: 2 in, 2 out]
        n195 = String Length(string=w291) -> (length=w290:i32)
        n196 = Equal To 0?(x=w290) -> (x = 0?=w289:bool)
        n197 = case shown="True" w289 {
          frame False {
          }
          frame True {
            n198 = One Button Dialog(message="A filename has not been entered!") -> ()  [unwired: 1 in, 1 out]
          }
        }
      }
      event "Stop Test": Value Change {
        n199 = event-data() -> ()  [unwired: 1 in, 6 out]
        n200 = flat-sequence {
          tunnel: w297 -> [w299]
          tunnel: [w299] -> w296
          tunnel: [w298] -> w294
          tunnel: w296 -> [w303]
          tunnel: [w302] -> w295
          tunnel: w294 -> [w302]
          tunnel: [w301] -> w293
          tunnel: w295 -> [w307]
          tunnel: w293 -> [w306]
          tunnel: [T11."Disabled and Grayed Out" ("Disabled")] -> _
          frame #0 {
            n201 = local read "Connected?"() -> (w298:bool)
            n202 = local write "Stop Cmd"(T1 1.0 ("Stop Cmd")) -> ()
          }
          frame #1 {
            n203 = Enqueue Element(queue=w303, element=Control_3."main" ("Enum")) -> (queue out=w301:refnum<queue>)  [unwired: 2 in, 2 out]
          }
          frame #2 {
            n204 = case shown="True" w307 {
              tunnel: w306 -> [w308 w311]
              tunnel: [w308 w310] -> _
              frame False {
              }
              frame True {
                n205 = local write "Connected?"(FALSE ("Connected?")) -> ()
                n206 = Enqueue Element(queue=w311, element=Control_3."Multigas disconnect" ("Enum")) -> (queue out=w310:refnum<queue>)  [unwired: 2 in, 2 out]
              }
            }
          }
        }
      }
      event "Stopped?": Value Change {
        n207 = event-data() -> ()  [unwired: 1 in, 5 out]
        n208 = flat-sequence {
          tunnel: w315 -> [w319]
          tunnel: [w318] -> w314
          tunnel: [w317] -> w313
          tunnel: w314 -> [w321]
          tunnel: w313 -> [w320]
          frame #0 {
            n209 = local read "Connected?"() -> (w317:bool)
            n210 = Enqueue Element(queue=w319, element=Control_3."main" ("Enum")) -> (queue out=w318:refnum<queue>)  [unwired: 2 in, 2 out]
          }
          frame #1 {
            n211 = case shown="True" w320 {
              tunnel: w321 -> [_ w322]
              frame False {
              }
              frame True {
                n212 = local write "Connected?"(FALSE ("Connected?")) -> ()
                n213 = Enqueue Element(queue=w322, element=Control_3."Multigas disconnect" ("Enum")) -> ()  [unwired: 2 in, 3 out]
              }
            }
          }
        }
      }
      event "Alarm ack": Value Change {
        # "system alarm - set to off"
        n214 = event-data() -> ()  [unwired: 1 in, 5 out]
        n215 = local write "Acknowledge"(TRUE ("Acknowledge")) -> ()
        n216 = property on="Soft Alarm" class="Bool (strict)"("Value"=FALSE ("Acknowledge")) -> ()  [unwired: 2 in, 2 out]
        n217 = property on="Alarm ack" class="Bool"("DisabledEnum"=T11."Disabled and Grayed Out" ("Disabled")) -> ()  [unwired: 2 in, 2 out]
      }
      event "Purge System": Value Change {
        n218 = event-data() -> ()  [unwired: 1 in, 5 out]
        n219 = flat-sequence {
          tunnel: w329 -> [w331]
          tunnel: [w331] -> w328
          tunnel: w328 -> [w332]
          frame #0 {
            n220 = local write "Enum 1"(u16 4 ("Test number")) -> ()
          }
          frame #1 {
            n221 = Enqueue Element(queue=w332, element=Control_3."start test" ("Enum")) -> ()  [unwired: 2 in, 3 out]
          }
        }
      }
      event "Clear log": Value Change {
        n222 = event-data() -> ()  [unwired: 1 in, 5 out]
        n223 = local write "Table"(string[][] [] ("Table")) -> ()
      }
      event "Adv Settings": Value Change {
        # "To be updated"
        # "SO2 conc\nNOx conc\nCO conc\nHC conc\nBleed ratio N2\nBleed ratio CO2"
        n224 = event-data() -> ()  [unwired: 1 in, 6 out]
        n225 = call "Advanced settings MAX.vi"() -> ("output cluster"=→"output cluster":T2)  [unwired: 1 in]
      }
    }
    "stop 2" <- w40
  }
  n226 = node-c288(nitl_modes."Discard missed periods, maintain original phase" ("Mode")) -> (w10:T12)  [unwired: 4 in]
  n227 = node-c288() -> (w3:T12)  [unwired: 4 in]
  n228 = timed-loop {
    timing: w10 -> [_]
    timing-out: [_] -> w9
    shift-right: [w458] -> _
    shift-left: path "" -> [w424]
    shift-right: [w517] -> _
    shift-left: w4 -> [w553]
    shift-right: [w459] -> _
    shift-left: _ -> [w528]
    shift-right: [w507] -> _
    shift-left: w4 -> [w510]
    shift-right: [w508] -> _
    shift-left: w4 -> [w509]
    shift-right: [w450] -> _
    shift-left: 0 ("t") -> [w449]
    shift-right: [w440] -> _
    shift-left: _ -> [w429]
    shift-right: [w439] -> _
    shift-left: _ -> [w430]
    shift-right: [w438] -> _
    shift-left: _ -> [w431]
    shift-right: [w437] -> _
    shift-left: _ -> [w432]
    shift-right: [w436] -> _
    shift-left: _ -> [w433]
    shift-right: [w435] -> _
    shift-left: _ -> [w434]
    shift-right: [w414] -> _
    shift-left: _ -> [w415]
    stop <- w552 stop-if-true
    w466 = 54321.0 ("y")
    # "Flow Rate Guide"
    # "Temperature Guide"
    # "0   Flow Rate 1\n1   Flow Rate 2\n     ECM 1\n     ECM 2\n2   CO2 U\n3   CO U\n4   HC U\n5   O2 U\n7   CO2 D\n8   CO D\n9   HC D\n10 O2 D\n12 TC1X\n13 TC2A\n14 TC3Y\n15 TC4B\n16 TC5\n17 TC6\n32 Venturi 1\n33 Venturi 2\n34 Tank\n35 Bearing 1\n36 Bearing 2\n38 Ex A\n39 Ex B\n40 Ex C\n41 Ex D\n     MFC Box\n42 Furnace 1\n43 Furnace 2\n44 NO 1 ?? \n45 Lambda 1\n46 NO 2 ??\n47 Lambda 2"
    n229 = node-c288() -> (→"Finished Late? [i-1]":bool, →"Iteration Duration":i64)  [unwired: 1 in, 1 out]
    n230 = shared-variable "RT CompactRIO Target 2\\Library 1.lvlib\\DATA"() -> (w551:dbl[])  [unwired: 1 in, 1 out]
    n231 = local read "MKS"() -> (w345:bool)
    n232 = Type Cast(type=w551, x=w551) -> (*(type *) &x=w561:dbl[])
    n233 = local read "Advanced Logging"() -> (w463:bool)
    n234 = Delete From Array(array=w561, length=4, index=0) -> (deleted portion=w558:dbl[], array with subset deleted=w340:dbl[])
    n235 = call "MKS.vi"("IP Address"="192.168.254.1", "Connect"=w345) -> ("Emissions"=w427:dbl[])  [unwired: 9 in]
    n236 = call "MKS.vi"("IP Address"="192.168.254.2", "Connect"=FALSE) -> ("Emissions"=w428:dbl[])  [unwired: 9 in]
    n237 = local read "Full system?"() -> (w457:bool)
    n238 = Index Array(array=w427, index=0) -> (element=w470:dbl)
    n239 = Index Array(array=w428, index=0) -> (element=w468:dbl)
    n240 = case shown="True" w463 {
      tunnel: [w658 w709] -> w464
      tunnel: w340 -> [w659 w709]
      tunnel: [w657 "Time\tFlow 1 g/s\tFlow 2 g/s\tECM 1\tECM 2\tTank Pressure\tTC1X\tTC2A\tTCY\tTC4B\tTC5\tTC6\tTC7\tTC8\tTC9\tTC10\tTC11\tTC12\tTC13\tTC14\tTC15\tTC16\tTC17\tTC18\tTC19\tTC20\tC Vent 1\tTC Vent 2\tTC Tank\tTC Fan B1\tTC Fan B2\tTC Cab\tTC Ex A\tTC Ex B\tTC Ex C\tTC Ex D\tSpare\tTC Furn 1\tTC Furn 2\tRapidox\tCO2 U %\tCO U %\tHC U ppm\tO2 U %\tNO U ppm\tCO2 D %\tCO D %\tHC D ppm\tO2 D %\tNO D ppm\tSwitch\tUEGO 1\tUEGO 2\tUEGO 3\tUEGO 4\tNOx Can 1\tNOx Can 2" ("Heading string 2")] -> w462
      tunnel: w457 -> [w656 _]
      frame False {
        n241 = case shown="True" w656 {
          tunnel: w659 -> [w674 w689]
          tunnel: [w665 w691] -> w658
          tunnel: ["Time\tFlow 1 g/s\tCO2 U %\tCO U %\tHC U ppm\tO2 U %\tNO U ppm\tCO2 D %\tCO D %\tHC D ppm\tO2 D %\tNO D ppm\tTC1X\tTC2A\tTCY\tTC4B\tTC5\tTC6\tTC7\tTC8\tRapidox\tLambda 1\tLambda 2\tNOX 1 ppm\tNOX 2 ppm\tUEGO 1\tUEGO 2" ("Heading string 2") "Time\tFlow 1 g/s\tFlow 2 g/s\tCO2 U %\tCO U %\tHC U ppm\tO2 U %\tNO U ppm\tCO2 D %\tCO D %\tHC D ppm\tO2 D %\tNO D ppm\tTC1X\tTC2A\tTCY\tTC4B\tTC5\tTC6\tTC7\tTC8\tRapidox\tLambda 1\tLambda 2\tNOX 1 ppm\tNOX 2 ppm\tUEGO 1\tUEGO 2" ("Heading string 2")] -> w657
          frame False {
            n242 = Delete From Array(array=w674, length=21, index=0) -> (deleted portion=w661:dbl[], array with subset deleted=w673:dbl[])
            n243 = Index Array(array=w673, index #1=47 ("index"), index #2=48 ("index"), index #3=49 ("index"), index #4=50 ("index"), index #5=51 ("index"), index #6=52 ("index"), index #7=53 ("index")) -> (element #1=w672:dbl, element #2=w671:dbl, element #3=w670:dbl, element #4=w669:dbl, element #5=w668:dbl, element #6=w667:dbl, element #7=w666:dbl)
            n244 = Delete From Array(array=w661, length=1, index=2) -> (array with subset deleted=w660:dbl[])  [unwired: 1 out]
            n245 = Build Array (concatenate)(w660, w672, w671, w670, w669, w668, w667, w666) -> (w665:dbl[])
          }
          frame True {
            n246 = Delete From Array(array=w689, length=21, index=0) -> (deleted portion=w686:dbl[], array with subset deleted=w690:dbl[])
            n247 = Index Array(array=w690, index #1=47 ("index"), index #2=48 ("index"), index #3=49 ("index"), index #4=50 ("index"), index #5=51 ("index"), index #6=52 ("index"), index #7=53 ("index")) -> (element #1=w698:dbl, element #2=w697:dbl, element #3=w696:dbl, element #4=w695:dbl, element #5=w694:dbl, element #6=w693:dbl, element #7=w692:dbl)
            n248 = Delete From Array(array=w686, length=2, index=1) -> (array with subset deleted=w684:dbl[])  [unwired: 1 out]
            n249 = Build Array (concatenate)(w684, w698, w697, w696, w695, w694, w693, w692) -> (w691:dbl[])
          }
        }
      }
      frame True {
        (unwired) "Time\tFlow 1 g/s\tFlow 2 g/s\tECM AFR\tCO2 U %\tCO U %\tHC U ppm\tO2 U %\tNO U ppm\tCO2 D %\tCO D %\tHC D ppm\tO2 D %\tNO D ppm\tTC1X\tTC2A\tTCY\tTC4B\tTC5\tTC6\tTC7\tTC8\tTC9\tTC10\tTC11\tTC12\tTC13\tTC14\tTC15\tTC16\tTC17\tTC18\tTC19\tTC20\tTC Vent 1\tTC Vent 2\tTC Fan B1\tTC Fan B2\tTC Cab\tTC Ex A\tTC Ex B\tTC Ex C\tTC Ex D\tTC Furn 1\tTC Furn 2\tNOX 1 ppm\tNLambda 1\tNOX 2 ppm\tNLambda 2\tEGO 1\tEGO 2\tEGO 3\tEGO 4\tCO2 U %\tCO U %\tHC U ppm\tO2 U %\tNO U ppm\tCO2 D %\tCO D %\tHC D ppm\tO2 D %\tNO D ppm\r\n" ("Heading string 2")
      }
    }
    n250 = Not Equal?(x=w470, y=w466) -> (x != y?=w469:bool)
    n251 = Not Equal?(x=w466, y=w468) -> (x != y?=w467:bool)
    n252 = Index Array(array=w558) -> (element #1=w459:dbl, element #2=w531:dbl, element #3=w343:dbl, element #4=w527:dbl)  [unwired: 4 in]
    "Error" <- w343
    n253 = case shown="False" w469 {
      tunnel: [w715 w726] -> w425
      tunnel: w428 -> [w714 w725]
      tunnel: w427 -> [_ w724]
      tunnel: w467 -> [w713 w723]
      tunnel: [w712 w720] -> w465
      frame False {
        n254 = case shown="False" w713 {
          tunnel: [dbl[] [54321.0] w719] -> w715
          tunnel: w714 -> [_ w719]
          tunnel: ["\r\n" ("Heading string 2") "\tNO\tNO2 (150)\tNO2 (2000)\tN2O\tNH3 (300)\tNH3 (3000)\tHNCO (400)\tH2O\tCO2\tCO (500)\tCO (1)\tCH4 (250)\tCH4 (3000)\tNOxP\tPropane\r\n" ("Heading string 2")] -> w710
          frame False {
          }
          frame True {
          }
        }
        n255 = Build Array(" " ("Heading string 2"), w710) -> (w712:string[])
      }
      frame True {
        n256 = case shown="True" w723 {
          tunnel: [w728 w732] -> w726
          tunnel: w725 -> [_ w731]
          tunnel: w724 -> [w728 w730]
          tunnel: ["\rn" ("Heading string 2") "\tNO\tNO2 (150)\tNO2 (2000)\tN2O\tNH3 (300)\tNH3 (3000)\tHNCO (400)\tH2O\tCO2\tCO (500)\tCO (1)\tCH4 (250)\tCH4 (3000)\tNOxP\tPropane\r" ("Heading string 2")] -> w721
          frame False {
          }
          frame True {
            n257 = Build Array (concatenate)(w730, w731) -> (w732:dbl[])
          }
        }
        n258 = Build Array("\tNO\tNO2 (150)\tNO2 (2000)\tN2O\tNH3 (300)\tNH3 (3000)\tHNCO (400)\tH2O\tCO2\tCO (500)\tCO (1)\tCH4 (250)\tCH4 (3000)\tNOxP\tPropane" ("Heading string 2"), w721) -> (w720:string[])
      }
    }
    n259 = To Unsigned Long Integer(number=w527) -> (unsigned 32bit integer=w526:u32)
    n260 = Number To Boolean Array(number=w526) -> (Boolean array=w541:bool[])
    n261 = Index Array(array=w541) -> (element #2=w539:bool, element #3=w538:bool, element #4=w523:bool, element #5=→"ExtAnUp":bool, element #6=→"ExtAnDn":bool)  [unwired: 6 in, 1 out]
    "Extractor Fan On" <- w523
    n262 = case shown="False" "7170 Override" {
      tunnel: [w581 FALSE ("Connect")] -> w337
      frame False {
        n263 = local read "7170"() -> (w581:bool)
      }
      frame True {
      }
    }
    n264 = case shown="2" w531 {
      tunnel: [w752 TRUE FALSE] -> w530
      tunnel: [w753 FALSE TRUE] -> w529
      frame 0, Default {
        n265 = local read "Pass"() -> (w753:bool)
        n266 = local read "Fail"() -> (w752:bool)
      }
      frame 1 {
      }
      frame 2 {
      }
    }
    "Pass" <- w529
    "Fail" <- w530
    n267 = Or(x=w539, y=w538) -> (x .or. y?=→"Doors Open":bool)
    n268 = Not(x=w523) -> (.not. x?=→"Doors Unlocked":bool)
    n269 = Less?(x=w459, y=w528) -> (x < y?=w525:bool)
    n270 = Path To String(path="File Path") -> (string=w521:string)
    n271 = local read "Connected"() -> (w524:bool)
    n272 = Concatenate Strings(w521, "\\" ("string"), "File Name") -> (w473:string)
    n273 = call "Mexa_7170.vi"("String 1 In"=w433, "Connect"=w337, "connection ID 1 In"=w432, "error out 1 In"=w431, "connection ID 2 In"=w430, "error out 2 In"=w429, "Time In"=w434) -> ("Emissions"=w426:dbl[], "String 1 Out"=w436:string, "connection ID 1 Out"=w437:refnum<k5>, "error 1 out"=w438:errorcluster, "connection ID 2 Out"=w439:refnum<k16>, "Time Out"=w435:i16, "error 2 out"=w440:errorcluster)  [unwired: 2 in]
    "Emissions" <- w426
    n274 = Build Array (concatenate)(w426, w425) -> (w338:dbl[])
    n275 = And(x=w524, y=w525) -> (x .and. y?=w516:bool)
    n276 = Build Array (concatenate)(w340, w338) -> (w339:dbl[])
    n277 = local write "Stopped?"(w516) -> ()
    n278 = Equal To 0?(x=w343) -> (x = 0?=w461:bool)
    n279 = Equal To 0?(x=w459) -> (x = 0?=w460:bool)
    n280 = Build Array (concatenate)(w464, w338) -> (w554:dbl[])
    n281 = Equal?(x=w459, y=2.0) -> (x = y?=w481:bool)
    n282 = String To Path(string=w473) -> (path=w518:path)
    n283 = Build Array(w461, w460) -> (w536:bool[])
    n284 = Equal?(x=w459, y=3.0) -> (x = y?=w478:bool)
    n285 = Equal?(x=w459, y=4.0) -> (x = y?=w476:bool)
    n286 = Boolean Array To Number(Boolean array=w536) -> (number=w535:u32)
    n287 = Index Array(array=w339, index=4) -> (element=→"Pressure":dbl)
    n288 = Not Equal?(x=w518, y=w424) -> (x != y?=w563:bool)
    n289 = Compound Arithmetic op=OR(w481, w478, w476) -> (w480:bool)
    n290 = case shown="2" w535 {
      tunnel: [w777 w778 w783 w785] -> _
      tunnel: [w777 w778 w783 w785] -> w534
      tunnel: [w777 w778 w783 w785] -> w533
      tunnel: [w777 w778 w781 w785] -> w532
      tunnel: [T11."Enabled" ("Disabled") T11."Enabled" ("Disabled") w781 w785] -> _
      tunnel: [FALSE FALSE FALSE TRUE] -> w515
      frame 0, Default {
        w777 = T11."Disabled and Grayed Out" ("Disabled")
      }
      frame 1 {
        w778 = T11."Disabled and Grayed Out" ("Disabled")
      }
      frame 2 {
        w781 = T11."Enabled" ("Disabled")
        w783 = T11."Disabled and Grayed Out" ("Disabled")
      }
      frame 3 {
        w785 = T11."Enabled" ("Disabled")
        (unwired) T11."Disabled and Grayed Out" ("Disabled")
      }
    }
    n291 = local read "Log Test Data"() -> (w474:bool)
    n292 = for {
      tunnel: w554 -> [w793] mode=indexing
      tunnel: [w792] -> w565 mode=indexing
      n293 = Number To Fractional String(number=w793, precision (6)=i16 3) -> (F-format string=w792:string)  [unwired: 2 in]
    }
    n294 = Select(t=w518, s=w563, f=w424) -> (s? t:f=w564:path)
    n295 = And(x=w474, y=w480) -> (x .and. y?=w580:bool)
    "Log?" <- w580
    n296 = case shown="True" w563 {
      tunnel: w564 -> [w786 w791]
      tunnel: [w786 w790] -> w562
      tunnel: w465 -> [_ w788]
      tunnel: w462 -> [_ w787]
      frame False {
      }
      frame True {
        # "setting up the header"
        n297 = Build Array (concatenate)(w787, w788) -> (w789:string[])
        n298 = call-poly <vilib>:"Write To Spreadsheet File.vi"("1D data"=w789, "file path (dialog if empty)"=w791) -> ("new file path (Not A Path if cancelled)"=w790:path)  [unwired: 6 in]
      }
    }
    n299 = Equal?(x=w459, y=0.0) -> (x = y?=w504:bool)
    n300 = case shown="5" w459 {
      tunnel: [w739 w742 w744 w746 TRUE FALSE] -> w354
      tunnel: [w739 TRUE TRUE TRUE w748 w750] -> w352
      tunnel: [TRUE w742 w744 w746 w748 w750] -> w351
      frame 0, Default {
        w739 = FALSE
      }
      frame 1 {
        w742 = FALSE
      }
      frame 2 {
        w744 = FALSE
      }
      frame 3 {
        w746 = FALSE
      }
      frame 4 {
        w748 = FALSE
        n301 = local write "Stop Cmd"(T1 0.0 ("Stop Cmd")) -> ()
      }
      frame 5 {
        w750 = FALSE
      }
    }
    n302 = property on="Execute Leak Test Button" class="Bool"("DisabledEnum"=w534) -> ()  [unwired: 2 in, 2 out]
    n303 = property on="Compile Test Button" class="Bool"("DisabledEnum"=w533) -> ()  [unwired: 2 in, 2 out]
    n304 = property on="Purge System" class="Bool"("DisabledEnum"=w532) -> ()  [unwired: 2 in, 2 out]
    n305 = property class="VI"("Front Panel.Closeable"=w515) -> ()  [unwired: 2 in, 2 out]
    n306 = local read "Full system?"() -> (w505:bool)
    n307 = Index Array(array=w338, index #1=0 ("index"), index #2=1 ("index"), index #3=2 ("index"), index #4=3 ("index")) -> ()  [unwired: 4 out]
    n308 = Equal?(x=w343, y=1024.0) -> (x = y?=w341:bool)
    n309 = case shown="True" "Demo On" {
      tunnel: w354 -> [w587 _]
      tunnel: [w587 w589] -> w353
      tunnel: w352 -> [w586 _]
      tunnel: w351 -> [w585 _]
      tunnel: [w585 w589] -> w350
      tunnel: [w586 TRUE] -> w349
      frame False {
      }
      frame True {
        w589 = FALSE
      }
    }
    "Cool Down" <- w353
    "Test In Progress" <- w349
    "Standby" <- w350
    n310 = case shown="True" w341 {
      tunnel: w343 -> [w583 _]
      tunnel: [w583 0.0 ("Numeric")] -> w344
      frame False {
      }
      frame True {
      }
    }
    n311 = Build Array(w505, w504) -> (w506:bool[])
    n312 = Boolean Array To Number(Boolean array=w506) -> (number=w503:u32)
    n313 = call "Demo_Guide.vi"("Time In"=w415, "Temperature Sync"="Demo Sync", "Duration -1"="Duration -1", "TempGuide"="Demo On") -> ("Output array"=w390:dbl[], "Time out"=w414:i32)  [unwired: 6 in]
    n314 = Not Equal To 0?(x=w344) -> (x != 0?=w556:bool)
    n315 = Not Equal?(x=w344, y=w553) -> (x != y?=w555:bool)
    n316 = case shown="True" w580 {
      tunnel: w562 -> [w797 w805]
      tunnel: [w797 w817] -> w458
      tunnel: w565 -> [_ w813]
      tunnel: w510 -> [_ w806]
      tunnel: w509 -> [w796 w801]
      tunnel: [w796 w803] -> w508
      tunnel: [w795 w802] -> w507
      frame False {
        n317 = local read "Log interval (seconds)"() -> (w795:T1)
      }
      frame True {
        n318 = Get Date/Time In Seconds() -> (seconds since 1Jan1904=w814:timestamp)
        n319 = Decrement(x=w806) -> (x-1=w807:T1)
        n320 = Less Than 0?(x=w807) -> (x < 0?=w808:bool)
        n321 = Equal To 0?(x=w807) -> (x = 0?=w809:bool)
        n322 = Build Array(w808, w809) -> (w810:bool[])
        n323 = Path To String(path=w805) -> (string=w800:string)
        "File name" <- w800
        n324 = Format Date/Time String(time format string (%c)="%d/%m/%y %H:%M:%S", seconds (now)=w814) -> (date/time string=w815:string)  [unwired: 1 in]
        n325 = Boolean Array To Number(Boolean array=w810) -> (number=w811:u32)
        n326 = case shown="2" w811 {
          tunnel: w806 -> [w824 w825 _]
          tunnel: [w823 w825 w828] -> w802
          tunnel: w800 -> [w822 w827 w831]
          tunnel: [w819 w827 w829] -> w804
          tunnel: [w818 w826 w830] -> w803
          tunnel: w801 -> [w818 w826 w834]
          frame 0, Default {
            n327 = Number To Decimal String(number=w818) -> (decimal integer string=w820:string)  [unwired: 1 in]
            n328 = call <vilib>:"Space Constant.vi"() -> ("String"=w821:string)
            n329 = Decrement(x=w824) -> (x-1=w823:T1)
            n330 = Concatenate Strings(w822, w821, w820) -> (w819:string)
          }
          frame 1 {
          }
          frame 2 {
            n331 = Increment(x=w834) -> (x+1=w830:dbl)
            n332 = local read "Log interval (seconds)"() -> (w828:T1)
            n333 = Number To Decimal String(number=w830) -> (decimal integer string=w832:string)  [unwired: 1 in]
            n334 = call <vilib>:"Space Constant.vi"() -> ("String"=w833:string)
            n335 = Concatenate Strings(w831, w833, w832) -> (w829:string)
          }
        }
        n336 = Build Array (concatenate)(w815, w813) -> (w799:string[])
        n337 = String To Path(string=w804) -> (path=w798:path)
        n338 = call-poly <vilib>:"Write To Spreadsheet File.vi"("append to file? (new file:F)"=TRUE, "1D data"=w799, "file path (dialog if empty)"=w798) -> ("new file path (Not A Path if cancelled)"=w817:path)  [unwired: 5 in]
      }
    }
    n339 = And(x=w556, y=w555) -> (x .and. y?=w557:bool)
    n340 = Index Array(array=w339, index #1=0 ("index"), index #2=1 ("index"), index #3=58 ("index"), index #4=55 ("index"), index #5=42 ("index"), index #6=44 ("index"), index #7=45 ("index"), index #8=47 ("index"), index #9=60 ("index"), index #10=46 ("index"), index #11=5 ("index"), index #12=6 ("index"), index #13=7 ("index"), index #14=8 ("index"), index #15=9 ("index"), index #16=10 ("index"), index #17=25 ("index"), index #18=26 ("index"), index #19=27 ("index"), index #20=28 ("index"), index #21=29 ("index"), index #22=31 ("index"), index #23=32 ("index"), index #24=33 ("index"), index #25=34 ("index"), index #26=36 ("index"), index #27=37 ("index"), index #28=43 ("index"), index #29=48 ("index"), index #30=45 ("index"), index #31=46 ("index"), index #32=2 ("index"), index #33=3 ("index")) -> (element #1=w452:dbl, element #2=w451:dbl, element #3=w413:dbl, element #4=w411:dbl, element #5=w409:dbl, element #6=w408:dbl, element #7=w407:dbl, element #8=w406:dbl, element #9=w405:dbl, element #10=w403:dbl, element #11=w402:dbl, element #12=w400:dbl, element #13=w398:dbl, element #14=w396:dbl, element #15=w394:dbl, element #16=w392:dbl, element #17=w385:dbl, element #18=w383:dbl, element #19=w381:dbl, element #20=w379:dbl, element #21=w377:dbl, element #22=w375:dbl, element #23=w373:dbl, element #24=w371:dbl, element #25=w369:dbl, element #26=→"Furnace temp 1":dbl, element #27=→"Furnace temp 2":dbl, element #28=w367:dbl, element #29=w365:dbl, element #30=w363:dbl, element #31=w361:dbl, element #32=w359:dbl, element #33=w357:dbl)
    n341 = case shown="True" w557 {
      tunnel: w344 -> [w759 w770]
      tunnel: w555 -> [w762 _]
      tunnel: [w758 w770] -> w517
      frame False {
        n342 = Equal To 0?(x=w759) -> (x = 0?=w763:bool)
        n343 = And(x=w763, y=w762) -> (x .and. y?=w761:bool)
        n344 = case shown="True" w761 {
          frame False {
          }
          frame True {
            w766 = FALSE ("Ack hard alarm!")
            n345 = property on="Hard Alarm" class="Bool (strict)"("Value"=w766) -> ()  [unwired: 2 in, 2 out]
            n346 = property on="System Alarm" class="Bool (strict)"("Value"=w766) -> ()  [unwired: 2 in, 2 out]
          }
        }
        n347 = case shown="False" "Acknowledge" {
          tunnel: [w764 0.0 ("Numeric")] -> w758
          tunnel: w759 -> [w764 _]
          frame False {
          }
          frame True {
          }
        }
      }
      frame True {
        n348 = local read "Table"() -> (w773:string[][])
        n349 = call "Error list.vi"("Error code"=w770, "Error array in"=w773) -> ("Hard alarm?"=w767:bool, "Error array out"=w772:string[][])  [unwired: 8 in]
        "Hard Alarm" <- w767
        "System Alarm" <- w767
        n350 = Not(x=w767) -> (.not. x?=w768:bool)
        "Soft Alarm" <- w768
        n351 = case shown="True" w768 {
          frame False {
          }
          frame True {
            n352 = property on="Alarm ack" class="Bool"("DisabledEnum"=T11."Enabled" ("Disabled")) -> ()  [unwired: 2 in, 2 out]
          }
        }
        n353 = local write "Table"(w772) -> ()
        n354 = local write "Acknowledge"(FALSE ("Acknowledge")) -> ()
        n355 = property on="Tab Control" class="TabCtl (strict)"("Value"=6) -> ()  [unwired: 2 in, 2 out]
      }
    }
    n356 = case shown="1" w503 {
      tunnel: w452 -> [w734 w736 _ _]
      tunnel: w451 -> [_ w735 _ _]
      tunnel: [w734 w736 w737 w738] -> w389
      tunnel: [0.0 ("y") w735 w737 w738] -> w387
      frame 0, Default {
      }
      frame 1 {
      }
      frame 2 {
        w737 = 0.0 ("y")
      }
      frame 3 {
        w738 = 0.0 ("y")
      }
    }
    n357 = case shown="False" "Demo On" {
      tunnel: w413 -> [w620 _]
      tunnel: [w620 w652] -> w412
      tunnel: w411 -> [w619 _]
      tunnel: [w619 w622] -> w410
      tunnel: w409 -> [w618 _]
      tunnel: [w618 w629] -> _
      tunnel: w408 -> [w617 _]
      tunnel: [w617 w629] -> _
      tunnel: w407 -> [w616 _]
      tunnel: [w616 w629] -> _
      tunnel: w406 -> [w615 _]
      tunnel: [w615 w629] -> _
      tunnel: [w614 w650] -> w404
      tunnel: w405 -> [w614 _]
      tunnel: w403 -> [w613 _]
      tunnel: [w613 w629] -> _
      tunnel: w402 -> [w612 _]
      tunnel: [w612 w648] -> w401
      tunnel: w400 -> [w611 _]
      tunnel: [w611 w646] -> w399
      tunnel: w398 -> [w610 _]
      tunnel: [w610 w629] -> w397
      tunnel: w396 -> [w609 _]
      tunnel: [w609 w629] -> w395
      tunnel: w394 -> [w608 _]
      tunnel: [w608 w629] -> w393
      tunnel: w392 -> [w607 _]
      tunnel: [w607 w629] -> w391
      tunnel: w390 -> [_ w655]
      tunnel: w389 -> [w606 _]
      tunnel: [w606 w654] -> w388
      tunnel: w387 -> [w605 _]
      tunnel: [w605 w629] -> w386
      tunnel: w385 -> [w604 _]
      tunnel: [w604 w644] -> w384
      tunnel: w383 -> [w603 _]
      tunnel: [w603 w629] -> w382
      tunnel: w381 -> [w602 _]
      tunnel: [w602 w642] -> w380
      tunnel: w379 -> [w601 _]
      tunnel: [w601 w640] -> w378
      tunnel: w377 -> [w600 _]
      tunnel: [w600 w638] -> w376
      tunnel: w375 -> [w599 _]
      tunnel: [w599 w636] -> w374
      tunnel: w373 -> [w598 _]
      tunnel: [w598 w634] -> w372
      tunnel: w371 -> [w597 _]
      tunnel: [w597 w632] -> w370
      tunnel: w369 -> [w596 _]
      tunnel: [w596 w631] -> w368
      tunnel: w367 -> [w595 _]
      tunnel: [w595 w630] -> w366
      tunnel: w365 -> [w594 _]
      tunnel: [w594 w629] -> w364
      tunnel: w363 -> [w593 _]
      tunnel: [w593 w627] -> w362
      tunnel: w361 -> [w592 _]
      tunnel: [w592 w628] -> w360
      tunnel: w359 -> [w591 _]
      tunnel: [w591 w628] -> w358
      tunnel: w357 -> [w590 _]
      tunnel: [w590 w628] -> w356
      frame False {
      }
      frame True {
        w628 = 5.0 ("Numeric")
        w629 = 0.0 ("Numeric")
        n358 = Index Array(array=w655, index #1=2 ("index"), index #2=13 ("index"), index #3=14 ("index"), index #4=0 ("index"), index #5=1 ("index"), index #6=4 ("index"), index #7=5 ("index"), index #8=6 ("index"), index #9=7 ("index"), index #10=8 ("index"), index #11=9 ("index"), index #12=10 ("index"), index #13=11 ("index"), index #14=15 ("index"), index #15=3 ("index"), index #16=12 ("index")) -> (element #1=w654:dbl, element #2=w652:dbl, element #3=w650:dbl, element #4=w648:dbl, element #5=w646:dbl, element #6=w644:dbl, element #7=w642:dbl, element #8=w640:dbl, element #9=w638:dbl, element #10=w636:dbl, element #11=w634:dbl, element #12=w632:dbl, element #13=w631:dbl, element #14=w630:dbl, element #15=w627:dbl, element #16=w622:dbl)
      }
    }
    n359 = call "Flow_Guide-plot.vi"("Temperature Sync"="Flow Sync", "Temp Band % (e.g. 1%=1.01)"="Flow Band %", "Mean(Off)/Interval(On)"="Mean(Off)/Interval(On) 2", "Guide"="FlowGuide") -> ()  [unwired: 5 in, 3 out]
    n360 = Merge Signals(w404) -> (→"HC Concentration (ppm)":dynamicdata)
    n361 = Merge Signals(w384, w382, w380, w378, w376) -> (→"System Temperatures (°C)":dynamicdata)
    n362 = Merge Signals(w374, w372, w370, w368) -> (→"Heat Exchanger Temperatures (°C)":dynamicdata)
    n363 = Merge Signals(w366, w364) -> (→"NO Concentration (ppm)":dynamicdata)
    n364 = Merge Signals(w362, w360, w358, w356) -> (→"Lambda":dynamicdata)
    n365 = Merge Signals(w388, w386) -> (→"Flow Rate (g/s)":dynamicdata)
    n366 = Merge Signals(w412, w410) -> (→"O2/CO Concentration":dynamicdata)
    n367 = call "Temp_Guide-plot.vi"("Time In"=w449, "Temperature Sync"="Temperature Sync", "Temp Band % (e.g. 1%=1.01)"="Temp Band %", "Mean(Off)/Interval(On)"="Mean(Off)/Interval(On)", "TempGuide"="TempGuide") -> ("Graph 4"=w448:dbl, "Graph 3"=w447:dbl, "Graph 2"=w446:dbl, "Graph 1"=w445:dbl, "Time out"=w450:i32)  [unwired: 2 in]
    n368 = local read "stop 2"() -> (w552:bool)
    n369 = Merge Signals(w401, w399, w397, w395, w393, w391, w445, w446, w447, w448) -> (→"Sample Temperatures (°C)":dynamicdata)
    n370 = node-c288() -> ()  [unwired: 1 in, 1 out]
  }
  n371 = timed-loop {
    timing: w3 -> [_]
    timing-out: [_] -> w2
    stop <- _ stop-if-true
    n372 = node-c288() -> ()  [unwired: 1 in, 1 out]
    n373 = shared-variable "RT CompactRIO Target 2\\Library 1.lvlib\\DATA_2"() -> (w846:dbl[])  [unwired: 1 in, 1 out]
    n374 = Add(x=0 ("index"), y="MFC Number") -> (x+y=w848:i32)
    n375 = Add(x="MFC Number", y=8) -> (x+y=w847:i32)
    n376 = call "MKS.vi"("IP Address"="192.168.254.2" ("IP_ADD [127.0.0.1]"), "Connect"="MKS 5Hz") -> ("Emissions"=w839:dbl[])  [unwired: 9 in]
    n377 = Build Array (concatenate)(w846, w839) -> (w845:dbl[])
    n378 = for {
      tunnel: w845 -> [w870] mode=indexing
      tunnel: [w869] -> w856 mode=indexing
      n379 = Number To Fractional String(number=w870, precision (6)=i16 3) -> (F-format string=w869:string)  [unwired: 2 in]
    }
    n380 = Index Array(array=w846, index #1=w848, index #2=w847) -> (element #1=w853:dbl, element #2=w852:dbl)
    n381 = Get Date/Time In Seconds() -> (seconds since 1Jan1904=w859:timestamp)
    n382 = local read "File name"() -> (w863:string)
    n383 = Index Array(array=w839, index="HC Index") -> (element=→"MKS HC":dbl)
    n384 = Format Date/Time String(time format string (%c)="%d/%m/%y %H:%M:%S", seconds (now)=w859) -> (date/time string=w857:string)  [unwired: 1 in]
    n385 = Concatenate Strings(w863, "_MFC" ("string")) -> (w861:string)
    n386 = Build Array (concatenate)(w857, w856) -> (w855:string[])
    n387 = String To Path(string=w861) -> (path=w858:path)
    n388 = local read "Log?"() -> (w854:bool)
    n389 = case shown="True" w854 {
      tunnel: w858 -> [w864 w867]
      tunnel: [w864 w865] -> _
      tunnel: w855 -> [_ w866]
      frame False {
      }
      frame True {
        n390 = call-poly <vilib>:"Write To Spreadsheet File.vi"("append to file? (new file:F)"=TRUE, "1D data"=w866, "file path (dialog if empty)"=w867) -> ("new file path (Not A Path if cancelled)"=w865:path)  [unwired: 5 in]
      }
    }
    n391 = Merge Signals(w853, w852) -> (→"MFC Setpoint/Delivery":dynamicdata)
    n392 = node-c288() -> ()  [unwired: 1 in, 1 out]
  }
  n393 = while {
    tunnel: w38 -> [w878]
    tunnel: w22 -> [w876]
    tunnel: w24 -> [w875]
    tunnel: [FALSE ("stop 2")] -> w12
    stop <- w879 stop-if-true
    n394 = Dequeue Element(queue=w878) -> (element=w877:T10)  [unwired: 2 in, 3 out]
    n395 = case shown="\"main\", Default" w877 {
      tunnel: w876 -> [_ _ _ w934 w945 w981 w1015 _ _ _ _ _ _ _ w1378 _ _ _ _ _ _ _]
      tunnel: w875 -> [_ _ _ _ _ _ _ _ w1028 w1043 w1098 w1143 _ _ _ _ _ _ _ _ _ _]
      frame "main", Default {
        # "20"
        # "25"
        # "30"
        # "15"
        # "10"
        # "5"
        # "0"
        # "30"
        # "25"
        # "20"
        # "15"
        # "10"
        # "5"
        # "0"
        # "Output Cluster\n\n0 NOx Conc\n1 CO conc %\n2 HC conc %\n3 Bleed H2O \n4 Bleed CO2\n5 Bleed N2 \n6 lambda P\n7 lambda I\n8 lambda D\n9 purge duration\n10 Target furnace lambda\n11 HC reaction ct\n12 Full system\n13 Log interval\n14 MKS 1\n15 MKS 2"
        n396 = local read "output cluster"() -> (w908:T2)
        n397 = Unbundle(w908) -> ("NOx Concentration (ppm)"=w894:T1, "CO concentration %"=w893:T1, "HC concentration %"=w892:T1, "Bleed H2O %"=w891:T1, "Bleed CO2 %"=w890:T1, "Bleed N2 %"=w905:T1, "lambda P"=w904:T1, "lambda I"=w903:T1, "lambda D"=w906:T1, "Purge duration (seconds)"=w907:T1, "Target furnace lambda"=w899:T1, "HC reaction constant"=w898:T1, w900:i16, "Log interval (HRS)"=→"Log interval (seconds)":T1, w887:i16, w886:i16, "Advanced Logging"=→"Advanced Logging":bool, "Cycle Length (Hours)"=w884:T1, "Heat Load Control"=w883:bool, w881:T1[])
        n398 = local read "Test Flow Rate(g/s)"() -> (w920:T1)
        n399 = local read "Test number"() -> (w925:u16)
        n400 = local read "Inlet LAMBDA"() -> (w912:T1)
        n401 = local read "NO ppm Loff"() -> (w910:T1)
        n402 = local read "NO:CO Ratio"() -> (w909:T1)
        n403 = local read "Inlet O2 (%)"() -> (w911:T1)
        n404 = local read "Connected"() -> (w914:bool)
        n405 = Boolean To (0,1)(Boolean=w883) -> (0, 1=w882:i16)
        n406 = Boolean To (0,1)(Boolean=w914) -> (0, 1=w897:i16)
        n407 = Build Array (concatenate)("Stop Cmd", w925, w920, "Test Start Temperature (°C)", "Test Stop temperature (°C)", "Furnace Ramp Rate (°C/min)", w912, w911, "Inlet LAMBDA Rich", "Inlet LAMBDA Lean", "Inlet Temperature (°C)", "NO ppm SW", w910, w909, "Temperature Limit (°C)", w897, "Inlet temp Age", "Flow rate Age", w894, w893, w892, w891, w890, w905, w904, w903, w906, w907, w899, w898, w900, w884, w882, w881) -> (w916:T1[])
        n408 = Not Equal To 0?(x=w900) -> (x != 0?=→"Full system?":bool)
        n409 = shared-variable "RT CompactRIO Target 2\\Library 1.lvlib\\Control Variables"(w916) -> ()  [unwired: 1 in, 1 out]
        n410 = Not Equal To 0?(x=w887) -> (x != 0?=w888:bool)
        "7170" <- w888
        n411 = Not Equal To 0?(x=w886) -> (x != 0?=w880:bool)
        "MKS" <- w880
        n412 = Or(x=w888, y=w880) -> (x .or. y?=→"Connected":bool)
      }
      frame "start test" {
        w926 = FALSE
        n413 = property on="Pass" class="Bool (strict)"("Value"=w926) -> ()  [unwired: 2 in, 2 out]
        n414 = property on="Fail" class="Bool (strict)"("Value"=w926) -> ()  [unwired: 2 in, 2 out]
        n415 = local write "Pass"(w926) -> ()
        n416 = local write "Fail"(w926) -> ()
        n417 = shared-variable "RT CompactRIO Target 2\\Library 1.lvlib\\Enum 1"("Enum 1") -> ()  [unwired: 1 in, 1 out]
      }
      frame "clear table 1" {
        n418 = property on="Sub-Cycle Name" class="Str (strict)"("Value"="" ("Subcycle name")) -> ()  [unwired: 2 in, 2 out]
        n419 = local write "Flag1"(FALSE) -> ()
        n420 = local write "Sub-Cycle Pattern"(string[][] [["", "0", "", "", "", "", "", "", "", "", "", "", ""], ["", "", "", "", "", "", "", "", "", "", "", "", ""], ["", "", "", "", "", "", "", "", "", "", "", "", ""], ["", "", "", "", "", "", "", "", "", "", "", "", ""], ["", "", "", "", "", "", "", "", "", "", "", "", ""], ["", "", "", "", "", "", "", "", "", "", "", "", ""], ["", "", "", "", "", "", "", "", "", "", "", "", ""], ["", "", "", "", "", "", "", "", "", "", "", "", ""], ["", "", "", "", "", "", "", "", "", "", "", "", ""], ["", "", "", "", "", "", "", "", "", "", "", "", ""], ["", "", "", "", "", "", "", "", "", "", "", "", ""], ["", "", "", "", "", "", "", "", "", "", "", "", ""], ["", "", "", "", "", "", "", "", "", "", "", "", ""], ["", "", "", "", "", "", "", "", "", "", "", "", ""], ["", "", "", "", "", "", "", "", "", "", "", "", ""], ["", "", "", "", "", "", "", "", "", "", "", "", ""], ["", "", "", "", "", "", "", "", "", "", "", "", ""], ["", "", "", "", "", "", "", "", "", "", "", "", ""], ["", "", "", "", "", "", "", "", "", "", "", "", ""], ["", "", "", "", "", "", "", "", "", "", "", "", ""], ["", "", "", "", "", "", "", "", "", "", "", "", ""], ["", "", "", "", "", "", "", "", "", "", "", "", ""], ["", "", "", "", "", "", "", "", "", "", "", "", ""], ["", "", "", "", "", "", "", "", "", "", "", "", ""], ["", "", "", "", "", "", "", "", "", "", "", "", ""], ["", "", "", "", "", "", "", "", "", "", "", "", ""], ["", "", "", "", "", "", "", "", "", "", "", "", ""], ["", "", "", "", "", "", "", "", "", "", "", "", ""], ["", "", "", "", "", "", "", "", "", "", "", "", ""], ["", "", "", "", "", "", "", "", "", "", "", "", ""], ["", "", "", "", "", "", "", "", "", "", "", "", ""]]) -> ()
      }
      frame "update list 1" {
        n421 = String To Path(string=w934) -> (path=w933:path)
        n422 = List Folder(path=w933, pattern="*.eyes") -> (filenames=w932:string[])  [unwired: 2 in, 3 out]
        n423 = property on="Sub-Cycle List" class="LstBox (strict)"("Item Names"=w932) -> ()  [unwired: 2 in, 2 out]
      }
      frame "save subc" {
        w938 = ".eyes" ("string")
        n424 = local read "Sub-Cycle Name"() -> (w937:T5)
        n425 = String To Path(string=w945) -> (path=w950:path)
        n426 = Equal?(x=w937, y="") -> (x = y?=w942:bool)
        n427 = List Folder(path=w950, pattern="*.eyes" ("string")) -> (filenames=w949:string[])  [unwired: 2 in, 3 out]
        n428 = Concatenate Strings(w937, w938) -> (w936:string)
        n429 = Concatenate Strings(w945, w937, w938) -> (w951:string)
        n430 = Search 1D Array(1D array=w949, element=w936) -> (index of element=w948:i32)  [unwired: 1 in]
        n431 = case shown="True" w942 {
          tunnel: [TRUE FALSE] -> w941
          frame False {
          }
          frame True {
            n432 = One Button Dialog(message="Insert file name!") -> ()  [unwired: 1 in, 1 out]
          }
        }
        n433 = String To Path(string=w951) -> (path=w944:path)
        n434 = Equal?(x=w948, y=-1) -> (x = y?=w946:bool)
        n435 = case shown="False" w946 {
          selector: w946 -> [_ w957]
          tunnel: [w955 w957] -> w940
          frame False {
            n436 = Two Button Dialog(message="A file with this name already exists!\nDo you want to overwrite?") -> (T button?=w955:bool)  [unwired: 2 in]
          }
          frame True {
          }
        }
        n437 = And(x=w940, y=w941) -> (x .and. y?=w939:bool)
        n438 = case shown="True" w939 {
          tunnel: w944 -> [_ w962]
          frame False {
          }
          frame True {
            n439 = local read "Sub-Cycle Pattern"() -> (w961:string[][])
            n440 = call "Table check.vi"("Input table"=w961) -> ("Incomplete?"=w959:bool, "Length"=w960:i32)  [unwired: 9 in]
            n441 = case shown="False" w959 {
              tunnel: w961 -> [w970 _]
              tunnel: w962 -> [w969 _]
              tunnel: w960 -> [w968 _]
              tunnel: string[] [] -> [w967 _]
              frame False {
                n442 = for {
                  N: w968 -> [_]
                  tunnel: w970 -> [w977]
                  shift-right: [w974] -> w966
                  shift-left: w967 -> [w975]
                  i -> [w976]
                  n443 = Index Array(array=w977, index (row)=w976) -> (element=w973:string[])  [unwired: 1 in]
                  n444 = Delete From Array(array=w973, index=0) -> (array with subset deleted=w972:string[])  [unwired: 1 in, 1 out]
                  n445 = Build Array (concatenate)(w975, w972) -> (w974:string[])
                }
                n446 = Build Array (concatenate)("SubCycle Data File for EYECAT - do not modify", w966) -> (w964:string[])
                n447 = call-poly <vilib>:"Write To Spreadsheet File.vi"("1D data"=w964, "file path (dialog if empty)"=w969) -> ()  [unwired: 6 in, 1 out]
              }
              frame True {
                n448 = One Button Dialog(message="The table is incomplete!\nplease review and save again!") -> ()  [unwired: 1 in, 1 out]
              }
            }
            n449 = local write "Flag1"(FALSE) -> ()
          }
        }
      }
      frame "load subc" {
        n450 = local read "Flag1"() -> (w982:bool)
        n451 = case shown="True" w982 {
          tunnel: [w1009 w1011] -> w980
          tunnel: w981 -> [w1009 w1011]
          tunnel: [TRUE w1010] -> w979
          frame False {
          }
          frame True {
            n452 = Two Button Dialog(message="The table has been modified.\nDo you want to continue?") -> (T button?=w1010:bool)  [unwired: 2 in]
          }
        }
        n453 = case shown="True" w979 {
          tunnel: w980 -> [_ w986]
          frame False {
          }
          frame True {
            n454 = property on="Sub-Cycle List" class="LstBox (strict)"() -> ("Item Names"=w998:string[])  [unwired: 2 in, 2 out]
            n455 = Index Array(array=w998, index="Sub-Cycle List") -> (element=w985:string)
            n456 = Concatenate Strings(w986, w985) -> (w996:string)
            n457 = Search/Split String(string=w985, search string/char (-)=".") -> (substring before match=w983:string)  [unwired: 1 in, 2 out]
            n458 = local write "Sub-Cycle Name"(w983) -> ()
            n459 = String To Path(string=w996) -> (path=w995:path)
            n460 = call-poly <vilib>:"Read From Spreadsheet File.vi"("file path (dialog if empty)"=w995) -> ("first row"=w991:string[])  [unwired: 6 in, 4 out]
            n461 = Delete From Array(array=w991, length=1, index=0) -> (array with subset deleted=w988:string[])  [unwired: 1 out]
            n462 = Array Size(array=w988) -> (size(s)=w994:i32)
            n463 = Divide(x=w994, y=12) -> (x/y=w987:dbl)
            n464 = for {
              N: w987 -> [_]
              shift-right: [w1004] -> _
              shift-left: w988 -> [w1007]
              tunnel: [w1003] -> w992 mode=indexing
              i -> [w1002]
              n465 = Increment(x=w1002) -> (x+1=w1001:i32)
              n466 = Delete From Array(array=w1007, length=12, index=0) -> (deleted portion=w999:string[], array with subset deleted=w1004:string[])
              n467 = Number To Decimal String(number=w1001) -> (decimal integer string=w1000:string)  [unwired: 1 in]
              n468 = Build Array (concatenate)(w1000, w999) -> (w1003:string[])
            }
            n469 = local write "Sub-Cycle Pattern"(w992) -> ()
          }
        }
      }
      frame "delete subc" {
        n470 = Two Button Dialog(message="This operation will permanently delete this file!\nDo you want to continue?") -> (T button?=w1014:bool)  [unwired: 2 in]
        n471 = case shown="True" w1014 {
          tunnel: w1015 -> [_ w1020]
          frame False {
          }
          frame True {
            n472 = local read "Sub-Cycle List"() -> (w1017:i32)
            n473 = property on="Sub-Cycle List" class="LstBox (strict)"() -> ("Item Names"=w1018:string[])  [unwired: 2 in, 2 out]
            n474 = Index Array(array=w1018, index=w1017) -> (element=w1022:string)
            n475 = Concatenate Strings(w1020, w1022) -> (w1021:string)
            n476 = local write "Flag1"(FALSE) -> ()
            n477 = String To Path(string=w1021) -> (path=w1019:path)
            n478 = Delete(path (use dialog)=w1019) -> ()  [unwired: 4 in, 3 out]
          }
        }
      }
      frame "clear table 2" {
        n479 = property on="Cycle Name" class="Str (strict)"("Value"="" ("Subcycle name")) -> ()  [unwired: 2 in, 2 out]
        n480 = local write "Flag 2"(FALSE) -> ()
        n481 = local write "Cycle Pattern"(string[][] [["", "", "", "", ""], ["", "", "", "", ""], ["", "", "", "", ""], ["", "", "", "", ""], ["", "", "", "", ""], ["", "", "", "", ""], ["", "", "", "", ""], ["", "", "", "", ""], ["", "", "", "", ""], ["", "", "", "", ""], ["", "", "", "", ""], ["", "", "", "", ""], ["", "", "", "", ""], ["", "", "", "", ""], ["", "", "", "", ""], ["", "", "", "", ""], ["", "", "", "", ""], ["", "", "", "", ""], ["", "", "", "", ""], ["", "", "", "", ""], ["", "", "", "", ""], ["", "", "", "", ""], ["", "", "", "", ""], ["", "", "", "", ""], ["", "", "", "", ""], ["", "", "", "", ""], ["", "", "", "", ""], ["", "", "", "", ""], ["", "", "", "", ""], ["", "", "", "", ""], ["", "", "", "", ""]]) -> ()
      }
      frame "update list 2" {
        n482 = String To Path(string=w1028) -> (path=w1029:path)
        n483 = List Folder(path=w1029, pattern="*.eyec") -> (filenames=w1027:string[])  [unwired: 2 in, 3 out]
        n484 = property on="Cycle List" class="LstBox (strict)"("Item Names"=w1027) -> ()  [unwired: 2 in, 2 out]
      }
      frame "save cycle" {
        w1030 = ".eyec" ("string")
        n485 = local read "Cycle Name"() -> (w1031:T5)
        n486 = String To Path(string=w1043) -> (path=w1044:path)
        n487 = List Folder(path=w1044, pattern="*.eyec" ("string")) -> (filenames=w1042:string[])  [unwired: 2 in, 3 out]
        n488 = Equal?(x=w1031, y="") -> (x = y?=w1037:bool)
        n489 = Concatenate Strings(w1031, w1030) -> (w1033:string)
        n490 = Search 1D Array(1D array=w1042, element=w1033) -> (index of element=w1041:i32)  [unwired: 1 in]
        n491 = Concatenate Strings(w1043, w1031, w1030) -> (w1046:string)
        n492 = case shown="True" w1037 {
          tunnel: [TRUE FALSE] -> w1035
          frame False {
          }
          frame True {
            n493 = One Button Dialog(message="Insert file name!") -> ()  [unwired: 1 in, 1 out]
          }
        }
        n494 = String To Path(string=w1046) -> (path=w1045:path)
        n495 = Equal?(x=w1041, y=-1) -> (x = y?=w1039:bool)
        n496 = case shown="False" w1039 {
          selector: w1039 -> [_ w1095]
          tunnel: [w1093 w1095] -> w1036
          frame False {
            n497 = Two Button Dialog(message="A file with this name already exists!\nDo you want to overwrite?") -> (T button?=w1093:bool)  [unwired: 2 in]
          }
          frame True {
          }
        }
        n498 = And(x=w1036, y=w1035) -> (x .and. y?=w1034:bool)
        n499 = case shown="True" w1034 {
          tunnel: w1045 -> [_ w1053]
          frame False {
          }
          frame True {
            n500 = local read "Cycle Pattern"() -> (w1052:string[][])
            n501 = call "Table check.vi"("Input table"=w1052) -> ("Incomplete?"=w1050:bool, "Length"=w1051:i32)  [unwired: 9 in]
            n502 = case shown="False" w1050 {
              tunnel: w1053 -> [w1062 _]
              tunnel: w1052 -> [w1061 _]
              tunnel: w1051 -> [w1054 _]
              frame False {
                n503 = Number To Decimal String(number=w1054) -> (decimal integer string=w1057:string)  [unwired: 1 in]
                n504 = for {
                  N: w1054 -> [_]
                  tunnel: w1061 -> [w1091]
                  shift-right: [w1079] -> w1058
                  shift-left: string[] [] -> [w1089]
                  i -> [w1090]
                  w1070 = 12 ("length")
                  n505 = Index Array(array=w1091, index (row)=w1090) -> (element=w1085:string[])  [unwired: 1 in]
                  n506 = Index Array(array=w1085, index=3) -> (element=w1075:string)
                  n507 = Index Array(array=w1085, index=1) -> (element=w1074:string)
                  n508 = Concatenate Strings("C:\\Setup Files\\Subcycles Folder\\", w1074) -> (w1086:string)
                  n509 = String To Path(string=w1086) -> (path=w1087:path)
                  n510 = call-poly <vilib>:"Read From Spreadsheet File.vi"("file path (dialog if empty)"=w1087) -> ("first row"=w1078:string[])  [unwired: 6 in, 4 out]
                  n511 = Delete From Array(array=w1078, length=1, index=0) -> (array with subset deleted=w1072:string[])  [unwired: 1 out]
                  n512 = String Length(string=w1072) -> (length=w1081:i32[])
                  n513 = Array Size(array=w1081) -> (size(s)=w1073:i32)
                  n514 = Divide(x=w1073, y=w1070) -> (x/y=w1071:dbl)
                  n515 = Decrement(x=w1071) -> (x-1=w1063:dbl)
                  n516 = Multiply(x=w1070, y=w1063) -> (x*y=w1069:dbl)
                  n517 = Number To Decimal String(number=w1063) -> (decimal integer string=w1080:string)  [unwired: 1 in]
                  n518 = Delete From Array(array=w1072, length=12, index=w1069) -> (deleted portion=w1066:string[], array with subset deleted=w1067:string[])
                  n519 = Index Array(array=w1066, index=0) -> (element=w1064:string)
                  n520 = Build Array (concatenate)(w1074, w1075, w1080, w1064, w1067) -> (w1084:string[])
                  n521 = Build Array (concatenate)(w1089, w1084) -> (w1079:string[])
                }
                n522 = local write "Flag 2"(FALSE) -> ()
                n523 = Build Array (concatenate)("Cycle Data File for EYECAT - do not modify", w1057, w1058) -> (w1059:string[])
                n524 = call-poly <vilib>:"Write To Spreadsheet File.vi"("1D data"=w1059, "file path (dialog if empty)"=w1062) -> ()  [unwired: 6 in, 1 out]
              }
              frame True {
                n525 = One Button Dialog(message="The table is incomplete!\nplease review and save again!") -> ()  [unwired: 1 in, 1 out]
              }
            }
          }
        }
      }
      frame "load cycle" {
        n526 = local read "Flag 2"() -> (w1099:bool)
        n527 = case shown="True" w1099 {
          tunnel: [w1138 w1140] -> w1096
          tunnel: w1098 -> [w1138 w1140]
          tunnel: [TRUE ("T button?") w1139] -> w1097
          frame False {
          }
          frame True {
            n528 = Two Button Dialog(message="The table has been modified.\nDo you want to continue?") -> (T button?=w1139:bool)  [unwired: 2 in]
          }
        }
        n529 = case shown="True" w1097 {
          tunnel: w1096 -> [_ w1102]
          frame False {
          }
          frame True {
            n530 = property on="Cycle List" class="LstBox (strict)"() -> ("Item Names"=w1118:string[])  [unwired: 2 in, 2 out]
            n531 = Index Array(array=w1118, index="Cycle List") -> (element=w1104:string)
            n532 = Concatenate Strings(w1102, w1104) -> (w1117:string)
            n533 = Search/Split String(string=w1104, search string/char (-)=".") -> (substring before match=w1103:string)  [unwired: 1 in, 2 out]
            n534 = String To Path(string=w1117) -> (path=w1116:path)
            n535 = local write "Cycle Name"(w1103) -> ()
            n536 = call-poly <vilib>:"Read From Spreadsheet File.vi"("file path (dialog if empty)"=w1116) -> ("first row"=w1100:string[])  [unwired: 6 in, 4 out]
            n537 = Delete From Array(array=w1100, length=2, index=0) -> (array with subset deleted=w1101:string[])  [unwired: 1 out]
            n538 = Index Array(array=w1100, index=1) -> (element=w1115:string)
            n539 = Decimal String To Number(string=w1115) -> (number=w1114:i32)  [unwired: 2 in, 1 out]
            n540 = for {
              N: w1114 -> [_]
              tunnel: w1101 -> [w1136]
              tunnel: [w1131] -> w1109 mode=indexing
              shift-right: [w1121] -> _
              shift-left: 0 ("x") -> [w1122]
              i -> [w1135]
              w1132 = ""
              n541 = Increment(x=w1122) -> (x+1=w1120:i32)
              n542 = Increment(x=w1120) -> (x+1=w1128:i32)
              n543 = Increment(x=w1135) -> (x+1=w1130:i32)
              n544 = Number To Decimal String(number=w1130) -> (decimal integer string=w1129:string)  [unwired: 1 in]
              n545 = Index Array(array=w1136, index #1=w1122, index #2=w1120, index #3=w1128) -> (element #1=w1134:string, element #2=w1133:string, element #3=w1127:string)
              n546 = Build Array(w1129, w1134, w1132, w1133, w1132) -> (w1131:string[])
              n547 = Decimal String To Number(string=w1127) -> (number=w1126:i32)  [unwired: 2 in, 1 out]
              n548 = Multiply(x=w1126, y=12 ("x")) -> (x*y=w1124:i32)
              n549 = Compound Arithmetic op=ADD(w1124, 4, w1122) -> (w1121:i32)
            }
            n550 = Insert Into Array(array=string[][] [["", "", "", "", ""], ["", "", "", "", ""], ["", "", "", "", ""], ["", "", "", "", ""], ["", "", "", "", ""], ["", "", "", "", ""], ["", "", "", "", ""], ["", "", "", "", ""], ["", "", "", "", ""], ["", "", "", "", ""], ["", "", "", "", ""], ["", "", "", "", ""], ["", "", "", "", ""], ["", "", "", "", ""], ["", "", "", "", ""], ["", "", "", "", ""], ["", "", "", "", ""], ["", "", "", "", ""], ["", "", "", "", ""], ["", "", "", "", ""], ["", "", "", "", ""], ["", "", "", "", ""], ["", "", "", "", ""], ["", "", "", "", ""], ["", "", "", "", ""], ["", "", "", "", ""], ["", "", "", "", ""], ["", "", "", "", ""], ["", "", "", "", ""], ["", "", "", "", ""], ["", "", "", "", ""]], index (row)=0, new element=w1109) -> (w1108:string[][])  [unwired: 1 in]
            n551 = local write "Cycle Pattern"(w1108) -> ()
          }
        }
      }
      frame "delete cycle" {
        n552 = Two Button Dialog(message="This operation will permanently delete this file!\nDo you want to continue?") -> (T button?=w1144:bool)  [unwired: 2 in]
        n553 = case shown="True" w1144 {
          tunnel: w1143 -> [_ w1149]
          frame False {
          }
          frame True {
            n554 = local read "Cycle List"() -> (w1150:i32)
            n555 = property on="Cycle List" class="LstBox (strict)"() -> ("Item Names"=w1151:string[])  [unwired: 2 in, 2 out]
            n556 = Index Array(array=w1151, index=w1150) -> (element=w1148:string)
            n557 = Concatenate Strings(w1149, w1148) -> (w1147:string)
            n558 = String To Path(string=w1147) -> (path=w1146:path)
            n559 = Delete(path (use dialog)=w1146) -> ()  [unwired: 4 in, 3 out]
            n560 = local write "Flag 2"(FALSE) -> ()
          }
        }
      }
      frame "calc HC CO" {
        n561 = local read "Sub-Cycle Pattern"() -> (w1168:string[][])
        n562 = Index Array(array=w1168, index (col) #1=3 ("disabled index (col)"), index (col) #2=4 ("index (col)"), index (col) #3=11 ("index (col)")) -> (element #1=w1158:string[], element #2=w1165:string[], element #3=w1152:string[])  [unwired: 3 in]
        n563 = Array Size(array=w1158) -> (size(s)=w1156:i32)
        n564 = Search 1D Array(1D array=w1158, element="") -> (index of element=w1155:i32)  [unwired: 1 in]
        n565 = Equal?(x=w1155, y=-1) -> (x = y?=w1157:bool)
        n566 = Select(t=w1156, s=w1157, f=w1155) -> (s? t:f=w1154:i32)
        n567 = for {
          N: w1154 -> [_]
          tunnel: [w1179] -> w1162 mode=indexing
          tunnel: [w1178] -> w1161 mode=indexing
          tunnel: w1158 -> [w1177] mode=indexing
          tunnel: w1165 -> [w1176] mode=indexing
          tunnel: w1152 -> [w1175] mode=indexing
          w1174 = ""
          n568 = Not Equal?(x=w1177, y=w1174) -> (x != y?=w1173:bool)
          n569 = Not Equal?(x=w1176, y=w1174) -> (x != y?=w1172:bool)
          n570 = Not Equal?(x=w1175, y=w1174) -> (x != y?=w1171:bool)
          n571 = Compound Arithmetic op=AND(w1173, w1172, w1171) -> (w1170:bool)
          n572 = case shown="True" w1170 {
            tunnel: w1177 -> [_ w1208]
            tunnel: w1176 -> [_ w1207]
            tunnel: [w1180 w1204] -> w1178
            tunnel: [w1180 w1203] -> w1179
            tunnel: w1175 -> [_ w1181]
            frame False {
              w1180 = ""
            }
            frame True {
              # "O2Eq"
              n573 = Fract/Exp String To Number(string=w1181) -> (number=w1182:dbl)  [unwired: 3 in, 1 out]
              n574 = Fract/Exp String To Number(string=w1208) -> (number=w1189:dbl)  [unwired: 3 in, 1 out]
              n575 = Fract/Exp String To Number(string=w1207) -> (number=w1185:dbl)  [unwired: 3 in, 1 out]
              n576 = Decrement(x=w1189) -> (x-1=w1190:dbl)
              n577 = Divide(x=w1182, y=20000.0) -> (x/y=w1183:dbl)
              n578 = Multiply(x=4.76, y=w1189) -> (x*y=w1194:dbl)
              n579 = Multiply(x=w1190, y=100.0) -> (x*y=w1192:dbl)
              n580 = Add(x=w1185, y=w1183) -> (x+y=w1186:dbl)
              n581 = Add(x=0.33, y=w1194) -> (x+y=w1196:dbl)
              n582 = Divide(x=w1192, y=w1196) -> (x/y=w1197:dbl)
              n583 = Subtract(x=w1186, y=w1197) -> (x-y=w1199:dbl)
              n584 = Multiply(x=w1199, y=2.0) -> (x*y=w1187:dbl)
              n585 = Divide(x=w1199, y=5.0) -> (x/y=w1188:dbl)
              n586 = Number To Fractional String(number=w1188, width (-)=i16 6, precision (6)=i16 3) -> (F-format string=w1203:string)  [unwired: 1 in]
              n587 = Number To Fractional String(number=w1187, width (-)=i16 6, precision (6)=i16 2) -> (F-format string=w1204:string)  [unwired: 1 in]
            }
          }
        }
        n588 = Replace Array Subset(array=w1168, new element #1=w1162, index (col) #1=5 ("disabled index (col)"), new element #2=w1161, index (col) #2=6 ("disabled index (col)")) -> (w1166:string[][])  [unwired: 2 in]
        n589 = local write "Sub-Cycle Pattern"(w1166) -> ()
      }
      frame "Total time calc" {
        w1223 = i16 2 ("width (-)")
        w1230 = ":"
        n590 = local read "Cycle Pattern"() -> (w1237:string[][])
        n591 = Index Array(array=w1237, index (col)=4 ("disabled index (col)")) -> (element=w1210:string[])  [unwired: 1 in]
        n592 = Array Size(array=w1210) -> (size(s)=w1212:i32)
        n593 = Search 1D Array(1D array=w1210, element="") -> (index of element=w1211:i32)  [unwired: 1 in]
        n594 = Equal?(x=w1211, y=-1) -> (x = y?=w1213:bool)
        n595 = Select(t=w1212, s=w1213, f=w1211) -> (s? t:f=w1209:i32)
        n596 = for {
          N: w1209 -> [_]
          tunnel: w1210 -> [w1245] mode=indexing
          shift-right: [w1247] -> w1233
          shift-left: 0 -> [w1248]
          n597 = xnode "Match Regular Expression"("input string"=w1245, "regular expression"=":" ("search string/char (-)")) -> ("before match"=w1244:string, "after match"=w1241:string)  [unwired: 4 in, 3 out]
          n598 = Decimal String To Number(string=w1244) -> (number=w1243:i32)  [unwired: 2 in, 1 out]
          n599 = Decimal String To Number(string=w1241) -> (number=w1240:i32)  [unwired: 2 in, 1 out]
          n600 = Multiply(x=w1243, y=60) -> (x*y=w1239:i32)
          n601 = Add(x=w1239, y=w1240) -> (x+y=w1238:i32)
          n602 = Add(x=w1238, y=w1248) -> (x+y=w1247:i32)
        }
        n603 = local read "Total Number of Cycles"() -> (w1234:T1)
        n604 = Multiply(x=w1233, y=w1234) -> (x*y=w1229:T1)
        n605 = Quotient & Remainder(x=w1229, y=3600.0) -> (x-y*floor(x/y)=w1216:T1, floor(x/y)=w1226:T1)
        n606 = Quotient & Remainder(x=w1216, y=60.0) -> (x-y*floor(x/y)=w1224:T1, floor(x/y)=w1225:T1)
        n607 = Number To Decimal String(number=w1226) -> (decimal integer string=w1231:string)  [unwired: 1 in]
        n608 = Number To Decimal String(number=w1225, width (-)=w1223) -> (decimal integer string=w1227:string)
        n609 = Number To Decimal String(number=w1224, width (-)=w1223) -> (decimal integer string=w1222:string)
        n610 = Concatenate Strings(w1231, w1230, w1227, w1230, w1222) -> (w1221:string)
        n611 = call <vilib>:"Search and Replace Pattern.vi"("string"=w1221, "regular expression (\"\")"=" " ("replace string (\"\")"), "replace string (\"\")"="0" ("replace string (\"\")"), "replace all? (F)"=TRUE) -> ("result string"=→"Total Test Duration (hrs)":string)  [unwired: 1 in, 1 out]
      }
      frame "update Cycle pattern " {
        n612 = local read "Cycle Pattern"() -> (w1376:string[][])
        n613 = Index Array(array=w1376, index (col)=1 ("disabled index (col)")) -> (element=w1361:string[])  [unwired: 1 in]
        n614 = String To Path(string=w1378) -> (path=w1379:path)
        n615 = Array Size(array=w1361) -> (size(s)=w1364:i32)
        n616 = Search 1D Array(1D array=w1361, element="") -> (index of element=w1363:i32)  [unwired: 1 in]
        n617 = List Folder(path=w1379, pattern="*.eyes") -> (filenames=w1377:string[])  [unwired: 2 in, 3 out]
        n618 = Equal?(x=w1363, y=-1) -> (x = y?=w1365:bool)
        n619 = Select(t=w1364, s=w1365, f=w1363) -> (s? t:f=w1362:i32)
        n620 = for {
          N: w1362 -> [_]
          tunnel: w1376 -> [w1395] mode=indexing
          tunnel: w1378 -> [w1388]
          tunnel: [w1390] -> w1371 mode=indexing
          tunnel: [w1392] -> w1375 mode=indexing
          tunnel: [w1389] -> w1372 mode=indexing
          tunnel: w1377 -> [w1387]
          tunnel: [w1382] -> w1368 mode=indexing
          n621 = Index Array(array=w1395, index #1=1 ("index"), index #2=3 ("index")) -> (element #1=w1386:string, element #2=w1391:string)
          n622 = Search 1D Array(1D array=w1387, element=w1386) -> (index of element=w1385:i32)  [unwired: 1 in]
          n623 = Not Equal?(x=w1385, y=-1) -> (x != y?=w1383:bool)
          n624 = case shown="True" w1383 {
            tunnel: [w1399 w1413] -> w1392
            tunnel: w1391 -> [_ w1409]
            tunnel: [w1399 w1407] -> w1390
            tunnel: [w1399 w1406] -> w1389
            tunnel: w1388 -> [_ w1405]
            tunnel: w1386 -> [w1398 w1404]
            tunnel: [w1397 w1404] -> w1382
            frame False {
              w1399 = "N/A" ("String")
              n625 = Concatenate Strings(w1398, " - File NOT AVAILABLE !!!" ("string")) -> (w1397:string)
            }
            frame True {
              w1417 = i16 2 ("width (-)")
              n626 = Concatenate Strings(w1405, w1404) -> (w1435:string)
              n627 = String To Path(string=w1435) -> (path=w1434:path)
              n628 = call <vilib>:"Search and Replace Pattern.vi"("string"=w1409, "regular expression (\"\")"="[a-x ]" ("format string"), "replace string (\"\")"="", "replace all? (F)"=TRUE) -> ("result string"=w1406:string)  [unwired: 1 in, 1 out]
              n629 = call-poly <vilib>:"Read From Spreadsheet File.vi"("file path (dialog if empty)"=w1434) -> ("first row"=w1403:string[])  [unwired: 6 in, 4 out]
              n630 = Delete From Array(array=w1403, length=1, index=0) -> (array with subset deleted=w1402:string[])  [unwired: 1 out]
              n631 = Array Size(array=w1402) -> (size(s)=w1433:i32)
              n632 = Equal?(x=w1406, y="") -> (x = y?=w1421:bool)
              n633 = Subtract(x=w1433, y=12) -> (x-y=w1431:i32)
              n634 = Select(t="0", s=w1421, f=w1406) -> (s? t:f=w1420:string)
              n635 = Index Array(array=w1402, index=w1431) -> (element=w1407:string)
              n636 = Decimal String To Number(string=w1420) -> (number=w1430:i32)  [unwired: 2 in, 1 out]
              n637 = Decimal String To Number(string=w1407) -> (number=w1429:i32)  [unwired: 2 in, 1 out]
              n638 = Multiply(x=w1430, y=w1429) -> (x*y=w1428:i32)
              n639 = Quotient & Remainder(x=w1428, y=60) -> (x-y*floor(x/y)=w1426:i32, floor(x/y)=w1425:i32)
              n640 = Number To Decimal String(number=w1426, width (-)=w1417) -> (decimal integer string=w1423:string)
              n641 = Number To Decimal String(number=w1425, width (-)=w1417) -> (decimal integer string=w1422:string)
              n642 = Concatenate Strings(w1422, ":", w1423) -> (w1416:string)
              n643 = call <vilib>:"Search and Replace Pattern.vi"("string"=w1416, "regular expression (\"\")"=" " ("replace string (\"\")"), "replace string (\"\")"="0" ("replace string (\"\")"), "replace all? (F)"=TRUE) -> ("result string"=w1413:string)  [unwired: 1 in, 1 out]
            }
          }
        }
        n644 = Replace Array Subset(array=w1376, new element #1=w1368, index (col) #1=1 ("disabled index (col)"), new element #2=w1371, index (col) #2=2 ("disabled index (col)"), new element #3=w1372, index (col) #3=3 ("disabled index (col)"), new element #4=w1375, index (col) #4=4 ("disabled index (col)")) -> (w1380:string[][])  [unwired: 4 in]
        n645 = local write "Cycle Pattern"(w1380) -> ()
      }
      frame "load cycle name" {
        n646 = property on="Cycle Pattern" class="Tbl (strict)"() -> ("EditPos"=w1441:T3)  [unwired: 2 in, 2 out]
        n647 = Unbundle By Name(w1441) -> ("Row"=w1439:i32, "Column"=w1438:i32)
        n648 = local read "Cycle Pattern"() -> (w1437:string[][])
        n649 = call "SubCycles list.vi"() -> ("Subcycle name"=w1440:string)  [unwired: 10 in, 1 out]
        n650 = Replace Array Subset(array=w1437, new element=w1440, index (row)=w1439, index (col)=w1438) -> (w1436:string[][])
        n651 = local write "Cycle Pattern"(w1436) -> ()
      }
      frame "load test array" {
        n652 = local read "Total Test Duration (hrs)"() -> (w1449:T8)
        n653 = local read "Cycle Name"() -> (w1445:T5)
        n654 = Equal?(x=w1445, y="") -> (x = y?=w1444:bool)
        n655 = Not Equal?(x=w1449, y="0:00:00") -> (x != y?=w1443:bool)
        n656 = Or(x=w1443, y=w1444) -> (x .or. y?=w1442:bool)
        n657 = case shown="True" w1442 {
          selector: w1442 -> [w1450 _]
          tunnel: [FALSE TRUE] -> w1447
          frame False {
            n658 = case shown="False" w1450 {
              frame False {
                n659 = One Button Dialog(message="Incomplete Data!\nReview the cycle pattern!") -> ()  [unwired: 1 in, 1 out]
              }
              frame True {
              }
            }
          }
          frame True {
            w1456 = 0.0 ("default (0 I32)")
            n660 = local read "Cycle Name"() -> (w1471:T5)
            n661 = Concatenate Strings("C:\\Setup Files\\Cycles Folder\\", w1471, ".eyec" ("string")) -> (w1469:string)
            n662 = String To Path(string=w1469) -> (path=w1470:path)
            n663 = local read "Total Number of Cycles"() -> (w1467:T1)
            n664 = call-poly <vilib>:"Read From Spreadsheet File.vi"("file path (dialog if empty)"=w1470) -> ("first row"=w1453:string[])  [unwired: 6 in, 4 out]
            n665 = call "Remove names.vi"("Array in"=w1453) -> ("Array out"=w1462:string[])  [unwired: 10 in]
            n666 = Index Array(array=w1453, index #1=14 ("index"), index #2=15 ("index")) -> (element #1=w1458:string, element #2=w1454:string)
            n667 = Number To Decimal String(number="Ageing Gas") -> (decimal integer string=w1466:string)  [unwired: 1 in]
            n668 = Number To Decimal String(number=w1467) -> (decimal integer string=w1465:string)  [unwired: 1 in]
            n669 = Decimal String To Number(string=w1454, default (0L)=w1456) -> (number=w1455:dbl)  [unwired: 1 in, 1 out]
            n670 = Decimal String To Number(string=w1458, default (0L)=w1456) -> (number=w1457:dbl)  [unwired: 1 in, 1 out]
            n671 = property on="Inlet temp Age" class="DigNum (strict)"("Value"=w1457) -> ()  [unwired: 2 in, 2 out]
            n672 = property on="Flow rate Age" class="DigNum (strict)"("Value"=w1455) -> ()  [unwired: 2 in, 2 out]
            n673 = Build Array (concatenate)(w1466, w1465, w1462) -> (w1461:string[])
            n674 = shared-variable "RT CompactRIO Target 2\\Library 1.lvlib\\Ageing Variables"(w1461) -> ()  [unwired: 1 in, 1 out]
          }
        }
        "Test Compiled" <- w1447
      }
      frame "convert to num" {
        n675 = local read "EditPos Subc"() -> (w1476:T3)
        n676 = Unbundle By Name(w1476) -> ("Row"=w1477:i32, "Column"=w1474:i32)
        n677 = Equal?(x=w1474, y=7) -> (x = y?=w1473:bool)
        n678 = case shown="False" w1473 {
          tunnel: w1477 -> [_ w1482]
          tunnel: w1474 -> [_ w1480]
          tunnel: w1476 -> [_ _]
          frame True {
          }
          frame False {
            n679 = local read "Sub-Cycle Pattern"() -> (w1479:string[][])
            n680 = call "Conv to num.vi"("Column"=w1480, "Row"=w1482, "Array"=w1479) -> ("result string"=w1481:string)  [unwired: 8 in]
            n681 = Replace Array Subset(array=w1479, new element=w1481, index (row)=w1482, index (col)=w1480) -> (w1478:string[][])
            n682 = local write "Sub-Cycle Pattern"(w1478) -> ()
          }
        }
      }
      frame "check scycle name" {
        n683 = local read "Sub-Cycle Name"() -> (w1483:T5)
        n684 = call <vilib>:"Search and Replace Pattern.vi"("string"=w1483, "regular expression (\"\")"="[^0-9a-zA-Z ]" ("format string"), "replace string (\"\")"="", "replace all? (F)"=TRUE) -> ("result string"=w1489:string)  [unwired: 1 in, 1 out]
        n685 = Not Equal?(x=w1489, y=w1483) -> (x != y?=w1488:bool)
        n686 = case shown="False" w1488 {
          tunnel: w1489 -> [w1490 w1491]
          tunnel: [w1490 w1491] -> w1484
          frame False {
          }
          frame True {
            n687 = One Button Dialog(message="Unsuitable character for the file name!") -> ()  [unwired: 1 in, 1 out]
          }
        }
        n688 = local write "Sub-Cycle Name"(w1484) -> ()
      }
      frame "check cycle name" {
        n689 = local read "Cycle Name"() -> (w1493:T5)
        n690 = call <vilib>:"Search and Replace Pattern.vi"("string"=w1493, "regular expression (\"\")"="[^0-9a-zA-Z ]" ("format string"), "replace string (\"\")"="", "replace all? (F)"=TRUE) -> ("result string"=w1499:string)  [unwired: 1 in, 1 out]
        n691 = Not Equal?(x=w1499, y=w1493) -> (x != y?=w1498:bool)
        n692 = case shown="False" w1498 {
          tunnel: w1499 -> [w1500 w1501]
          tunnel: [w1500 w1501] -> w1494
          frame False {
          }
          frame True {
            n693 = One Button Dialog(message="Unsuitable character for the file name!") -> ()  [unwired: 1 in, 1 out]
          }
        }
        n694 = local write "Cycle Name"(w1494) -> ()
      }
      frame "Multigas connect" {
        # "add here logic to verify the user requirements and the machine state\n0 - not connected\n1 - MKS1 & Ext An Up\n2 - MKS2 & Ext An Dn\n3 - MKS 1 & 2  & Ext An Up & Dn"
        n695 = flat-sequence {
          frame #0 {
            "Connected?" <- TRUE
          }
        }
      }
      frame "Multigas disconnect" {
      }
    }
    n696 = local read "stop 2"() -> (w879:bool)
  }
  n697 = node-c288(w2) -> ()  [unwired: 1 out]
  n698 = local write "stop 2"(w12) -> ()
  n699 = node-c288(w9) -> ()  [unwired: 1 out]
  "Table" <- string[][] [] ("Table")
